vi "Phi Theta Scanning w Action Engine.vi"() -> ()   [LabVIEW 2022 SP3]
uses:
  C:/Users/mnopl/OneDrive/Documents/PhiThetaScanning/Thorlabs.MotionControl.Controls.dll
  Thorlabs.MotionControl.Controls.dll
  ActionEngineEnum.ctl
  <vilib>/DAQmx/read.llb/DAQmx Read (Analog 1D DBL 1Chan NSamp).vi
  <vilib>/Analysis/baseanly.llb/Mean (DBL).vi
  <vilib>/DAQmx/read.llb/DAQmx Read (Analog 2D DBL NChan NSamp).vi
  <vilib>/DAQmx/miscellaneous.llb/DAQmx Fill In Error Info.vi
  <vilib>/Analysis/NI_AALBase.lvlib
panel:
  out "Time Left":dbl
  out "X Origin":dbl
  out "Y Origin":dbl
  in  "Move to Origin":bool
  in  "Notes":string
  in  "X Center":dbl
  in  "Y Center":dbl
  in  "Tab Control 2":enum32{"Input 1", "Input 2"}(tab)
  out "Line Scan":dbl[](graph)
  in  "Save Line graph":bool
  out "Line Scan 2":dbl[](graph)
  in  "Save Line graph 2":bool
  in  "Duel Input":bool
  in  "Tab Control":enum32{"Input 1", "Input 2"}(tab)
  out "Graph":dbl[][](graph)
  in  "Save Image":bool
  in  "Save Data":bool
  in  "Name of File":string
  in  "Move to Cursor":bool
  in  "Save Image 2":bool
  out "Graph 2":dbl[][](graph)
  in  "Move to Cursor 2":bool
  in  "Estimate number\nof samples":bool
  in  "Connection":bool
  in  "Settings Y":T1={"Step Size (mm)"=10.0, "Initial Position"=0.0, "Move Absolute/Relative Position"=0.0, "Step Delay (ms)"=0, "Velocity (mm/s)"=0.0, "Acceleration (mm/s^2)"=0.0} {"Step Size (mm)" min=0.00046 format="%.8f"}
  in  "Settings X":T1={"Step Size (mm)"=10.0, "Initial Position"=0.0, "Move Absolute/Relative Position"=0.0, "Step Delay (ms)"=0, "Velocity (mm/s)"=0.0, "Acceleration (mm/s^2)"=0.0} {"Step Size (mm)" min=0.00046 format="%.8f"}
  in  "Estimate X Step Size":bool
  in  "2D Flyover":bool
  in  "Flyover Y Linescan":bool
  in  "Update Vel/Acc":bool
  in  "Grid points":dbl=3000.0
  in  "Save Phi/Theta":bool
  in  "Move to Saved Pos":bool
  in  "Save Position":bool
  out "Y Pos 1":dbl
  out "X Pos 1":dbl
  out "return value":dbl[][](array[numeric])
  in  "Acceleration":dbl=10.0
  in  "Measures/Pixel":dbl=7.0
  in  "Flyover X Linescan":bool
  in  "Move Y":bool
  in  "Move X":bool
  in  "Y Step Size":dbl=1.0
  in  "X Step Size":dbl=1.0
  in  "Move to Y":bool
  in  "Move to X":bool
  in  "Y Move":dbl=1.0
  in  "X Move":dbl=1.0
  out "Y Line Scan":dbl[](array[numeric])=[-inf, -inf, -inf, -inf, -inf, -inf]
  out "X Line Scan":dbl[](array[numeric])=[-inf, -inf, -inf, -inf, -inf, -inf]
  out "Scan Type":string="Scan"
  in  "Y Line Scan":bool
  in  "Abort":bool
  in  "X Line Scan":bool
  out "(X,Y)":cluster{dbl, dbl}[][](array[cluster])
  out "Phi Theta Data":dbl[][](graph)
  in  "Convert to phi/theta":bool
  in  "Y Pos":dbl=0.899996795693412
  in  "X Pos":dbl=1.0
  in  "Read Position":bool
  out "array of values":dbl[][](array[numeric])=[[-inf, -inf, -inf, -inf, -inf, -inf], [-inf, -inf, -inf, -inf, -inf, -inf], [-inf, -inf, -inf, -inf, -inf, -inf], [-inf, -inf, -inf, -inf, -inf, -inf], [-inf, -inf, -inf, -inf, -inf, -inf], [-inf, -inf, -inf, -inf, -inf, -inf]]
  out "task out":refnum<k21>
  in  "physical channels":tag="Dev1/ai0"
  in  "number of samples":i32=10000
  in  "rate":dbl=250000.0
  in  "maximum value":dbl=5.0 format="%0.2f"
  in  "minimum value":dbl=-5.0 format="%0.2f"
  in  "Take Single Measurement":bool
  out "Done Mov?":bool=TRUE
  in  "Y Length":dbl=5.0
  in  "X Length":dbl=5.0
  in  "2D Scan":bool
  in  "Velocity":dbl=2.0
  in  "Move Y (in)":bool
  in  "Move X (in)":bool
  in  "Time to wait":dbl=251.0
  out "Time":i32=77055304
  in  "Y Step Size (in)":dbl=1.0
  in  "X Step Size (in)":dbl=1.0
  in  "X=T,Y=F":bool
  in  "Moving?":bool
  in  "Stop":bool
  in  "KCubeStepperControl Y":refnum<k24>(container)
  in  "KCubeStepperControl X":refnum<k24>(container)
  in  "SerialNumber X":string="26005279"
  in  "SerialNumber Y":string="26005327"
  in  "Set Vel/Acc":bool
  out "array of values 2":dbl[][](array[numeric])
  # "Internal Variables"
  # "Only works with the first input"
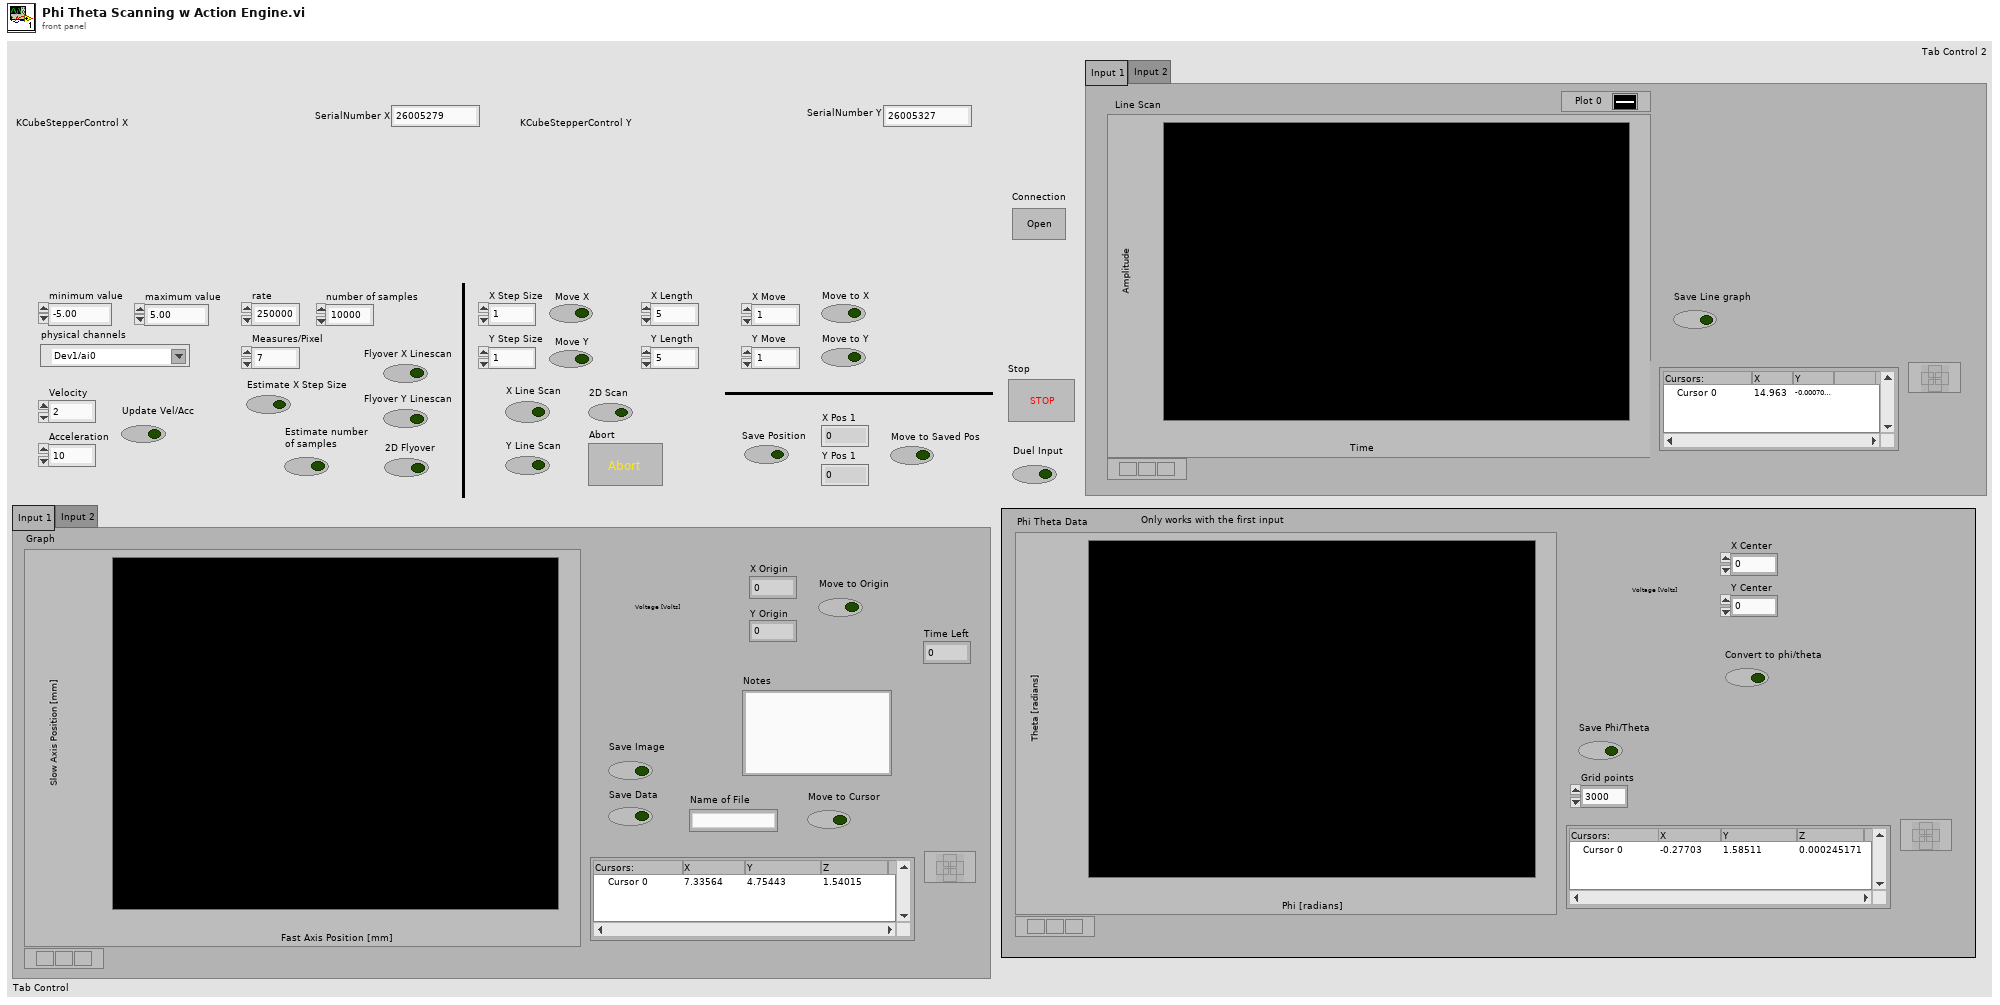
[diagram p1: front panel]
types:
  T1 = cluster{"Step Size (mm)":sgl, "Initial Position":dbl, "Move Absolute/Relative Position":dbl, "Step Delay (ms)":u32, "Velocity (mm/s)":dbl, "Acceleration (mm/s^2)":dbl}
  T2 = typedef "ActionEngineEnum.ctl" = enum16{"Open Connection", "Done", "Get Position", "Settings", "Home", "Move Absolute", "Move Relative", "Step", "Stop Action", "Close Connection"}
  T3 = typedef "LVPointDoubleTypeDef.ctl" = cluster{"Cursor X":dbl, "Cursor Y":dbl}
  T4 = typedef "imagedata.ctl" = cluster{"image type":i32, "image depth":i32, "image":u8[], "mask":u8[], "colors":u32[], "Rectangle":cluster{"left":i16, "top":i16, "right":i16, "bottom":i16}}
  T5 = cluster{"Y Step Size (in)":dbl, "Initial Position":dbl, "Move Absolute/Relative Position":dbl, "Step Delay (ms)":u32, "Velocity (mm/s)":dbl, "Acceleration (mm/s^2)":dbl}
  T6 = cluster{"X Step Size (in)":dbl, "Initial Position":dbl, "Move Absolute/Relative Position":dbl, "Step Delay (ms)":u32, "Velocity (mm/s)":dbl, "Acceleration (mm/s^2)":dbl}
  T7 = cluster{"Step Size (mm)":sgl, "Initial Position":dbl, "Move Absolute/Relative Position":dbl, "Step Delay (ms)":u32, "Velocity":dbl, "Acceleration":dbl}
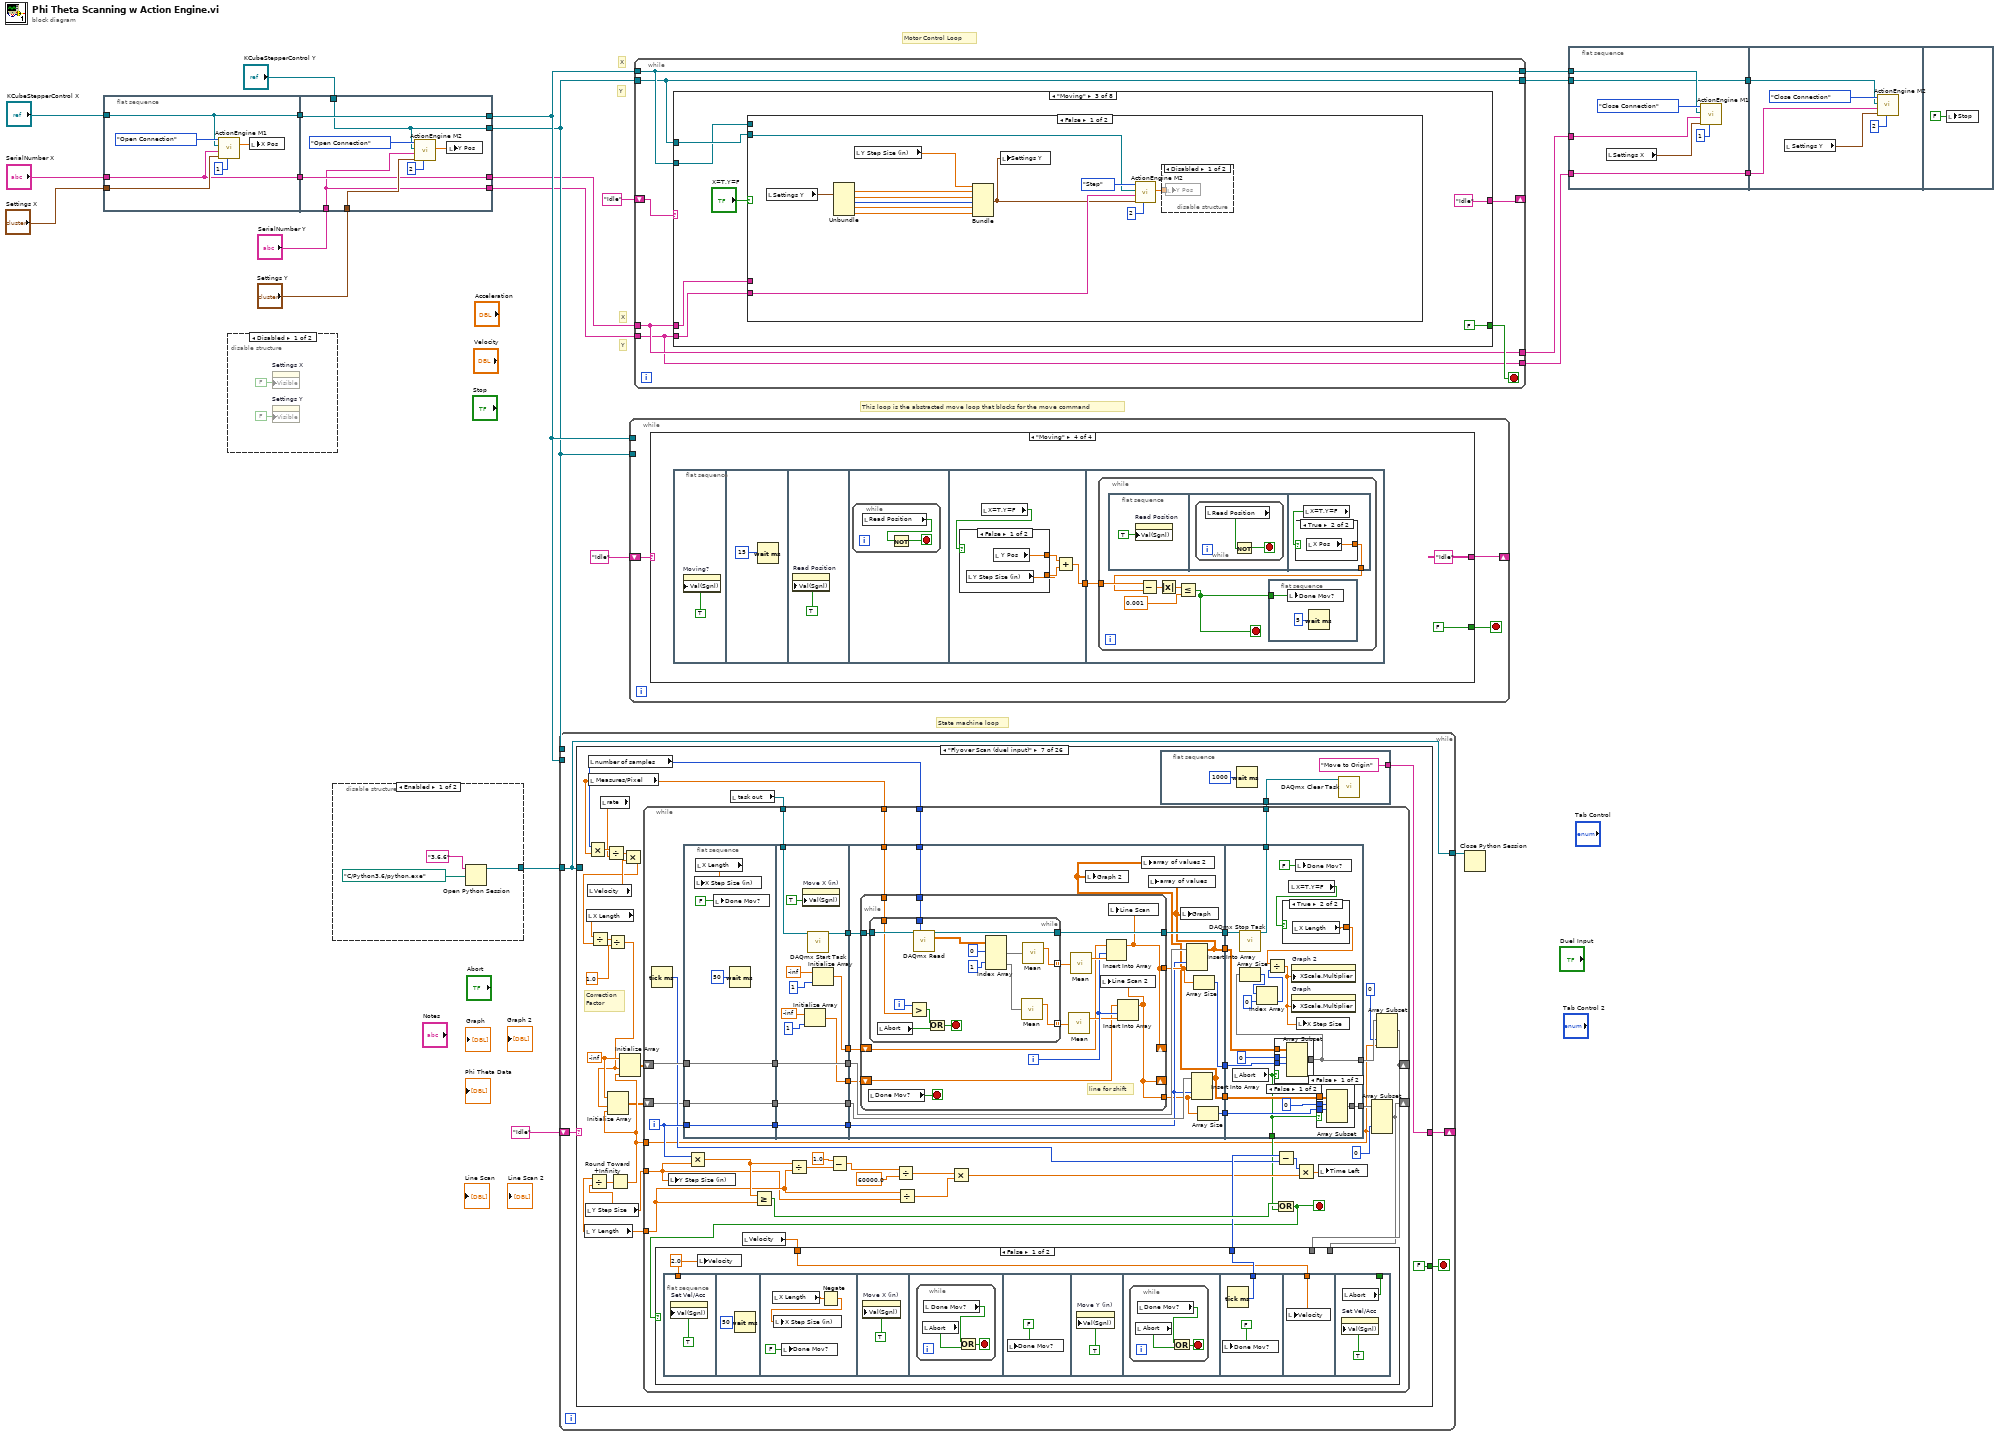
[diagram p0: block diagram]
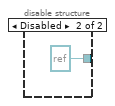
[diagram p3: hidden frame]
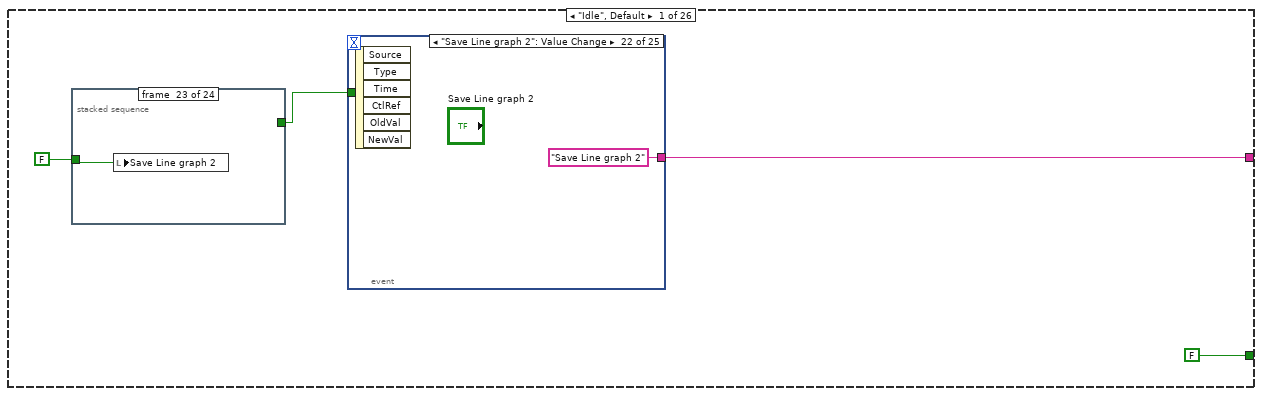
[diagram p4: hidden frame]
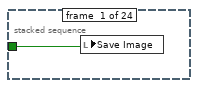
[diagram p5: hidden frame]
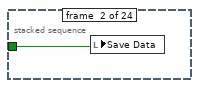
[diagram p6: hidden frame]
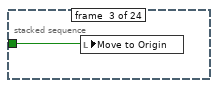
[diagram p7: hidden frame]
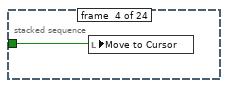
[diagram p8: hidden frame]
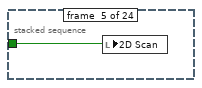
[diagram p9: hidden frame]
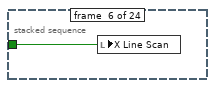
[diagram p10: hidden frame]
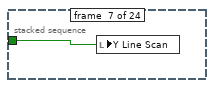
[diagram p11: hidden frame]
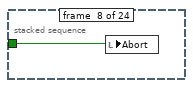
[diagram p12: hidden frame]
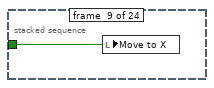
[diagram p13: hidden frame]
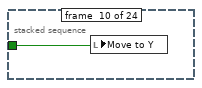
[diagram p14: hidden frame]
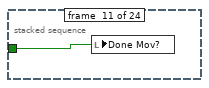
[diagram p15: hidden frame]
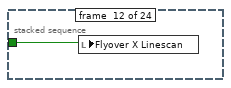
[diagram p16: hidden frame]
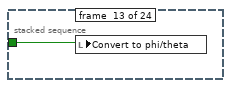
[diagram p17: hidden frame]
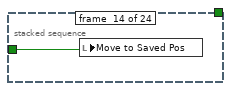
[diagram p18: hidden frame]
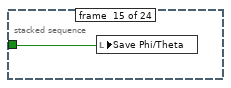
[diagram p19: hidden frame]
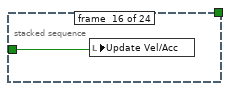
[diagram p20: hidden frame]
diagram:
  # "Y"
  # "X"
  # "State machine loop"
  # "Y"
  # "X"
  # "This loop is the abstracted move loop that blocks for the move command"
  # "Motor Control Loop"
  n1 = flat-sequence {
    tunnel: "SerialNumber X" -> [w24]
    tunnel: "Settings X" -> [w27]
    tunnel: "KCubeStepperControl X" -> [w25]
    tunnel: [w25] -> w10
    tunnel: [w24] -> w9
    tunnel: "SerialNumber Y" -> [w30]
    tunnel: "Settings Y" -> [w35]
    tunnel: "KCubeStepperControl Y" -> [w32]
    tunnel: w10 -> [w33]
    tunnel: w9 -> [w31]
    tunnel: [w33] -> w18
    tunnel: [w32] -> w17
    tunnel: [w31] -> w15
    tunnel: [w30] -> w16
    frame #0 {
      n2 = call "ActionEngine M1.vi"("ChannelNumber"=1, "Settings"=w27, "SerialNumber"=w24, "KCubeStepperControl"=w25, "Action"=ActionEngineEnum."Open Connection") -> ("Current Position"=w26:dbl)  [unwired: 4 in, 1 out]
      n3 = local write "X Pos"(w26) -> ()
    }
    frame #1 {
      n4 = call "ActionEngine M2.vi"("ChannelNumber"=2, "Settings"=w35, "SerialNumber"=w30, "KCubeStepperControl"=w32, "Action"=ActionEngineEnum."Open Connection") -> ("Current Position"=w34:dbl)  [unwired: 4 in, 1 out]
      n5 = local write "Y Pos"(w34) -> ()
    }
  }
  n6 = disable-structure shown="Disabled" {
    frame Disabled {
      n7 = property on="Settings X" class="Clust (strict)"("Visible"=FALSE) -> ()  [unwired: 2 in, 2 out]
      n8 = property on="Settings Y" class="Clust (strict)"("Visible"=FALSE) -> ()  [unwired: 2 in, 2 out]
    }
    frame Enabled {
    }
  }
  n9 = disable-structure shown="Enabled" {
    disable-tunnel: [w42 refnum<k35> refnum ("session out")] -> w20
    frame Enabled {
      n10 = Open Python Session(python version="3.6.6" ("Python version"), python path=path "C:/Python3.6/python.exe" ("Python path")) -> (session out=w42:refnum<k35>)  [unwired: 1 in, 1 out]
    }
    frame Disabled {
    }
  }
  n11 = while {
    shift-right: [w46] -> _
    shift-left: "Idle" -> [w47]
    tunnel: w20 -> [w44]
    tunnel: [w44] -> w19
    tunnel: w18 -> [_]
    tunnel: w17 -> [_]
    stop <- w45 stop-if-true
    n12 = case shown="\"Flyover Scan (duel input)\"" w47 {
      tunnel: [w51 "Init Graph" "Init Graph" ("Scan Type") w176 "Move to Origin" w543 w692 "Idle" ("Scan Type") "Idle" ("Scan Type") "Move to Origin" ("Scan Type") "Move to Origin" ("Scan Type") "Idle" ("Scan Type") "Idle" ("Scan Type") "Idle" "Idle" "Idle" ("Scan Type") "Idle" ("Scan Type") "Idle" "Idle" ("Scan Type") "Idle" "Idle" "Idle" ("Scan Type") "Idle" ("Scan Type") "Idle" ("Scan Type") "Idle" ("Scan Type") "Idle"] -> w46
      tunnel: [FALSE FALSE FALSE FALSE FALSE FALSE FALSE FALSE FALSE FALSE FALSE FALSE FALSE FALSE FALSE FALSE FALSE FALSE FALSE FALSE FALSE FALSE FALSE FALSE FALSE TRUE] -> w45
      tunnel: w44 -> [_ _ _ _ _ _ _ _ _ _ _ _ _ _ _ _ _ w1203 _ _ _ w1378 _ _ _ _]
      frame "Idle", Default {
        n13 = stacked-sequence {
          tunnel: FALSE -> [w52 w53 w54 w55 w56 w57 w58 w59 w60 w61 w62 w63 w64 w65 w66 w67 w68 w69 w70 w71 w72 w73 w74 w75]
          tunnel: [_ _ _ _ _ _ _ _ _ _ _ _ _ _ _ _ _ _ _ _ _ _ _ w75] -> w48
          frame #0 {
            n14 = local write "Save Image"(w52) -> ()
          }
          frame #1 {
            n15 = local write "Save Data"(w53) -> ()
          }
          frame #2 {
            n16 = local write "Move to Origin"(w54) -> ()
          }
          frame #3 {
            n17 = local write "Move to Cursor"(w55) -> ()
          }
          frame #4 {
            n18 = local write "2D Scan"(w56) -> ()
          }
          frame #5 {
            n19 = local write "X Line Scan"(w57) -> ()
          }
          frame #6 {
            n20 = local write "Y Line Scan"(w58) -> ()
          }
          frame #7 {
            n21 = local write "Abort"(w59) -> ()
          }
          frame #8 {
            n22 = local write "Move to X"(w60) -> ()
          }
          frame #9 {
            n23 = local write "Move to Y"(w61) -> ()
          }
          frame #10 {
            n24 = local write "Done Mov?"(w62) -> ()
          }
          frame #11 {
            n25 = local write "Flyover X Linescan"(w63) -> ()
          }
          frame #12 {
            n26 = local write "Convert to phi/theta"(w64) -> ()
          }
          frame #13 {
            n27 = local write "Move to Saved Pos"(w65) -> ()
          }
          frame #14 {
            n28 = local write "Save Phi/Theta"(w66) -> ()
          }
          frame #15 {
            n29 = local write "Update Vel/Acc"(w67) -> ()
          }
          frame #16 {
            n30 = local write "Flyover Y Linescan"(w68) -> ()
          }
          frame #17 {
            n31 = local write "2D Flyover"(w69) -> ()
          }
          frame #18 {
            n32 = local write "Estimate X Step Size"(w70) -> ()
          }
          frame #19 {
            n33 = local write "Estimate number\nof samples"(w71) -> ()
          }
          frame #20 {
            n34 = local write "Move to Cursor 2"(w72) -> ()
          }
          frame #21 {
            n35 = local write "Save Image 2"(w73) -> ()
          }
          frame #22 {
            n36 = local write "Save Line graph 2"(w74) -> ()
          }
          frame #23 {
            n37 = local write "Save Position"(w75) -> ()
          }
        }
        n38 = event shown="[21] \"Save Line graph 2\": Value Change" {
          selector: _ -> [_ _ _ _ _ _ _ _ _ _ _ _ _ _ _ _ _ _ _ _ _ _ _ _ _]
          dyn-events: _ -> [_ _ _ _ _ _ _ _ _ _ _ _ _ _ _ _ _ _ _ _ _ _ _ _ _]
          timeout: _ -> [_ _ _ _ _ _ _ _ _ _ _ _ _ _ _ _ _ _ _ _ _ _ _ _ _]
          tunnel: ["Idle" "Convert" "Move to Cursor" "Move to Cursor 2" "Stop" "Init Daq" "Init Daq (duel input)" "Move to Origin" "Move to Saved Position" "Init Daq" "Init Daq" "Init Daq" "Init Daq" "Move to" "Move to" "Update Vel/Acc" "Save Position" "Save Image" "Save Image 2" "Save Phi/Theta" "Save Line graph" "Save Line graph 2" "Save Data" "Estimate X Step Size" "Estimate number of samples"] -> w51
          tunnel: w48 -> [_ _ _ _ _ _ _ _ _ _ _ _ _ _ _ _ _ _ _ _ _ _ _ _ _]
          event Timeout {
            n39 = event-data() -> ()  [unwired: 1 in, 3 out]
          }
          event "Convert to phi/theta": Value Change {
            n40 = event-data() -> ()  [unwired: 1 in, 6 out]
          }
          event "Move to Cursor": Value Change {
            n41 = event-data() -> ()  [unwired: 1 in, 6 out]
          }
          event "Move to Cursor 2": Value Change {
            n42 = event-data() -> ()  [unwired: 1 in, 6 out]
          }
          event "Stop": Value Change {
            n43 = event-data() -> ()  [unwired: 1 in, 6 out]
          }
          event "2D Scan": Value Change {
            n44 = event-data() -> ()  [unwired: 1 in, 6 out]
            n45 = local read "X Step Size"() -> (w81:dbl)
            n46 = local read "Y Step Size"() -> (w82:dbl)
            n47 = local write "Scan Type"("Scan" ("Scan Type")) -> ()
            n48 = local write "Y Step Size (in)"(w82) -> ()
            n49 = local write "X Step Size (in)"(w81) -> ()
          }
          event "2D Flyover": Value Change {
            n50 = event-data() -> ()  [unwired: 1 in, 6 out]
            n51 = local read "Y Step Size"() -> (w87:dbl)
            n52 = local read "X Step Size"() -> (w88:dbl)
            n53 = local write "X Step Size (in)"(w88) -> ()
            n54 = local write "Y Step Size (in)"(w87) -> ()
            n55 = local write "Scan Type"("Flyover Scan (duel input)" ("Scan Type")) -> ()
          }
          event "Move to Origin": Value Change {
            n56 = event-data() -> ()  [unwired: 1 in, 6 out]
          }
          event "Move to Saved Pos": Value Change {
            n57 = event-data() -> ()  [unwired: 1 in, 6 out]
          }
          event "X Line Scan": Value Change {
            n58 = event-data() -> ()  [unwired: 1 in, 6 out]
            n59 = local read "X Step Size"() -> (w91:dbl)
            n60 = local write "X Step Size (in)"(w91) -> ()
            n61 = local write "Scan Type"("Line Scan" ("Scan Type")) -> ()
            n62 = local write "X=T,Y=F"(TRUE ("X=T,Y=F")) -> ()
          }
          event "Flyover X Linescan": Value Change {
            n63 = event-data() -> ()  [unwired: 1 in, 6 out]
            n64 = local read "X Step Size"() -> (w98:dbl)
            n65 = local write "X Step Size (in)"(w98) -> ()
            n66 = local write "Scan Type"("Flyover Linescan" ("Scan Type")) -> ()
            n67 = local write "X=T,Y=F"(TRUE ("X=T,Y=F")) -> ()
          }
          event "Flyover Y Linescan": Value Change {
            n68 = event-data() -> ()  [unwired: 1 in, 6 out]
            n69 = local read "Y Step Size"() -> (w100:dbl)
            n70 = local write "Y Step Size (in)"(w100) -> ()
            n71 = local write "Scan Type"("Flyover Linescan" ("Scan Type")) -> ()
            n72 = local write "X=T,Y=F"(FALSE ("X=T,Y=F")) -> ()
          }
          event "Y Line Scan": Value Change {
            n73 = event-data() -> ()  [unwired: 1 in, 6 out]
            n74 = local read "Y Step Size"() -> (w103:dbl)
            n75 = local write "Y Step Size (in)"(w103) -> ()
            n76 = local write "X=T,Y=F"(FALSE ("X=T,Y=F")) -> ()
            "Scan Type" <- "Line Scan" ("Scan Type")
          }
          event "Move to X": Value Change {
            n77 = event-data() -> ()  [unwired: 1 in, 6 out]
            n78 = local write "X=T,Y=F"(TRUE ("X=T,Y=F")) -> ()
          }
          event "Move to Y": Value Change {
            n79 = event-data() -> ()  [unwired: 1 in, 6 out]
            n80 = local write "X=T,Y=F"(FALSE ("X=T,Y=F")) -> ()
          }
          event "Update Vel/Acc": Value Change {
            n81 = event-data() -> ()  [unwired: 1 in, 6 out]
          }
          event "Save Position": Value Change {
            n82 = event-data() -> ()  [unwired: 1 in, 6 out]
          }
          event "Save Image": Value Change {
            n83 = event-data() -> ()  [unwired: 1 in, 6 out]
          }
          event "Save Image 2": Value Change {
            n84 = event-data() -> ()  [unwired: 1 in, 6 out]
          }
          event "Save Phi/Theta": Value Change {
            n85 = event-data() -> ()  [unwired: 1 in, 6 out]
          }
          event "Save Line graph": Value Change {
            n86 = event-data() -> ()  [unwired: 1 in, 6 out]
          }
          event "Save Line graph 2": Value Change {
            n87 = event-data() -> ()  [unwired: 1 in, 6 out]
          }
          event "Save Data": Value Change {
            n88 = event-data() -> ()  [unwired: 1 in, 6 out]
          }
          event "Estimate X Step Size": Value Change {
            n89 = event-data() -> ()  [unwired: 1 in, 6 out]
          }
          event "Estimate number\nof samples": Value Change {
            n90 = event-data() -> ()  [unwired: 1 in, 6 out]
          }
        }
      }
      frame "Init Daq" {
        w121 = -inf
        n91 = local read "Y Length"() -> (w134:dbl)
        n92 = local read "Y Step Size"() -> (w133:dbl)
        n93 = local read "X Length"() -> (w131:dbl)
        n94 = local read "X Step Size"() -> (w130:dbl)
        n95 = Divide(x=w134, y=w133) -> (x/y=w135:dbl)
        n96 = Divide(x=w131, y=w130) -> (x/y=w132:dbl)
        n97 = Round Toward +Infinity(x=w135) -> (ceil(x): smallest int >= x=w124:dbl)
        n98 = Round Toward +Infinity(x=w132) -> (ceil(x): smallest int >= x=w129:dbl)
        n99 = Increment(x=w124) -> (x+1=w122:dbl)
        n100 = Increment(x=w129) -> (x+1=w123:dbl)
        n101 = call "Initialize DAQ Assistant.vi"("minimum value"="minimum value", "maximum value"="maximum value", "rate"="rate", "number of samples"="number of samples", "physical channels"="physical channels") -> ("task out"=→"task out":refnum<k21>)  [unwired: 5 in, 1 out]
        n102 = Initialize Array(w121, w122) -> (→"Y Line Scan":dbl[])
        n103 = Initialize Array(w121, w123, w122) -> (→"array of values":dbl[][])
        n104 = Initialize Array(w121, w123) -> (→"X Line Scan":dbl[])
      }
      frame "Init Daq (duel input)" {
        w146 = -inf
        n105 = local read "Y Step Size"() -> (w158:dbl)
        n106 = local read "X Step Size"() -> (w161:dbl)
        n107 = local read "Y Length"() -> (w157:dbl)
        n108 = local read "X Length"() -> (w160:dbl)
        n109 = local read "number of samples"() -> (w149:i32)
        n110 = local read "physical channels"() -> (w150:tag)
        n111 = local read "maximum value"() -> (w151:dbl)
        n112 = local read "minimum value"() -> (w152:dbl)
        n113 = local read "rate"() -> (w148:dbl)
        n114 = Divide(x=w157, y=w158) -> (x/y=w156:dbl)
        n115 = Divide(x=w160, y=w161) -> (x/y=w159:dbl)
        n116 = Round Toward +Infinity(x=w156) -> (ceil(x): smallest int >= x=w163:dbl)
        n117 = Round Toward +Infinity(x=w159) -> (ceil(x): smallest int >= x=w162:dbl)
        n118 = Increment(x=w163) -> (x+1=w144:dbl)
        n119 = Increment(x=w162) -> (x+1=w145:dbl)
        n120 = call "Initialize DAQ Assistant (duel input).vi"("minimum value"=w152, "maximum value"=w151, "rate"=w148, "number of samples"=w149, "physical channels"=w150) -> ("task out"=w147:refnum<k21>)  [unwired: 5 in, 1 out]
        n121 = Initialize Array(w146, w145, w144) -> (→"array of values 2":dbl[][])
        n122 = Initialize Array(w146, w144) -> (w153:dbl[])
        n123 = Initialize Array(w146, w145, w144) -> (w154:dbl[][])
        n124 = Initialize Array(w146, w145) -> (w155:dbl[])
        n125 = local write "task out"(w147) -> ()
        n126 = local write "Y Line Scan"(w153) -> ()
        n127 = local write "array of values"(w154) -> ()
        n128 = local write "X Line Scan"(w155) -> ()
      }
      frame "Init Graph" {
        n129 = local read "Acceleration"() -> (w172:dbl)
        n130 = local read "Scan Type"() -> (w176:string)
        n131 = local read "Velocity"() -> (w173:dbl)
        n132 = flat-sequence {
          tunnel: [w261] -> w166
          tunnel: ["X Pos"] -> w178
          tunnel: ["Y Pos"] -> w177
          frame #0 {
            n133 = property on="Read Position" class="Bool (strict)"("Val(Sgnl)"=TRUE) -> ()  [unwired: 2 in, 2 out]
          }
          frame #1 {
            n134 = while {
              tunnel: [w262] -> w261
              stop <- w265 stop-if-true
              n135 = local read "Read Position"() -> (w264:bool)
              n136 = Not(x=w264) -> (.not. x?=w265:bool)
              n137 = Wait (ms)(milliseconds to wait=u32 10) -> (millisecond timer value=w262:u32)
            }
          }
          frame #2 {
            "X Origin" <- "X Pos"
            "Y Origin" <- "Y Pos"
          }
        }
        n138 = case shown="\"Flyover Scan\"" w176 {
          tunnel: [w194 w212 w228 w244] -> w170
          tunnel: w169 -> [w194 w212 w228 w244]
          frame "Line Scan", Default {
            n139 = local read "X=T,Y=F"() -> (w195:bool)
            n140 = case shown="False" w195 {
              frame False {
                n141 = flat-sequence {
                  frame #0 {
                    n142 = local read "Y Length"() -> (w197:dbl)
                    n143 = Divide(x=w197, y=2.0) -> (x/y=w198:dbl)
                    n144 = Negate(x=w198) -> (-x=w199:dbl)
                    n145 = local write "Y Step Size (in)"(w199) -> ()
                  }
                  frame #1 {
                    n146 = local write "Done Mov?"(FALSE ("Done Mov?")) -> ()
                    n147 = property on="Move Y (in)" class="Bool (strict)"("Val(Sgnl)"=TRUE ("Value (Signaling)")) -> ()  [unwired: 2 in, 2 out]
                  }
                  frame #2 {
                    n148 = while {
                      stop <- w202 stop-if-true
                      n149 = local read "Done Mov?"() -> (w202:bool)
                    }
                  }
                  frame #3 {
                    n150 = local write "Done Mov?"(FALSE ("Done Mov?")) -> ()
                  }
                }
              }
              frame True {
                n151 = flat-sequence {
                  frame #0 {
                    n152 = local read "X Length"() -> (w207:dbl)
                    n153 = Divide(x=w207, y=2.0) -> (x/y=w206:dbl)
                    n154 = Negate(x=w206) -> (-x=w205:dbl)
                    n155 = local write "X Step Size (in)"(w205) -> ()
                  }
                  frame #1 {
                    n156 = property on="Move X (in)" class="Bool (strict)"("Val(Sgnl)"=TRUE ("Value (Signaling)")) -> ()  [unwired: 2 in, 2 out]
                    n157 = local write "Done Mov?"(FALSE ("Done Mov?")) -> ()
                  }
                  frame #2 {
                    n158 = while {
                      stop <- w210 stop-if-true
                      n159 = local read "Done Mov?"() -> (w210:bool)
                    }
                  }
                  frame #3 {
                    n160 = local write "Done Mov?"(FALSE ("Done Mov?")) -> ()
                  }
                }
              }
            }
          }
          frame "Scan" {
            n161 = flat-sequence {
              frame #0 {
                n162 = local read "X Length"() -> (w220:dbl)
                n163 = local read "Y Length"() -> (w218:dbl)
                n164 = Divide(x=w220, y=2.0) -> (x/y=w216:dbl)
                n165 = Divide(x=w218, y=2.0) -> (x/y=w214:dbl)
                n166 = Negate(x=w216) -> (-x=w215:dbl)
                n167 = Negate(x=w214) -> (-x=w213:dbl)
                n168 = local write "X Step Size (in)"(w215) -> ()
                n169 = local write "Y Step Size (in)"(w213) -> ()
              }
              frame #1 {
                n170 = local write "Done Mov?"(FALSE ("Done Mov?")) -> ()
                n171 = property on="Move Y (in)" class="Bool (strict)"("Val(Sgnl)"=TRUE ("Value (Signaling)")) -> ()  [unwired: 2 in, 2 out]
              }
              frame #2 {
                n172 = while {
                  stop <- w223 stop-if-true
                  n173 = local read "Done Mov?"() -> (w223:bool)
                }
              }
              frame #3 {
                n174 = local write "Done Mov?"(FALSE ("Done Mov?")) -> ()
                n175 = property on="Move X (in)" class="Bool (strict)"("Val(Sgnl)"=TRUE ("Value (Signaling)")) -> ()  [unwired: 2 in, 2 out]
              }
              frame #4 {
                n176 = while {
                  stop <- w226 stop-if-true
                  n177 = local read "Done Mov?"() -> (w226:bool)
                }
              }
              frame #5 {
                n178 = local write "Done Mov?"(FALSE ("Done Mov?")) -> ()
              }
            }
          }
          frame "Flyover Scan" {
            n179 = flat-sequence {
              frame #0 {
                n180 = local read "X Length"() -> (w236:dbl)
                n181 = local read "Y Length"() -> (w234:dbl)
                n182 = Divide(x=w236, y=2.0) -> (x/y=w232:dbl)
                n183 = Divide(x=w234, y=2.0) -> (x/y=w230:dbl)
                n184 = Negate(x=w232) -> (-x=w231:dbl)
                n185 = Negate(x=w230) -> (-x=w229:dbl)
                n186 = local write "X Step Size (in)"(w231) -> ()
                n187 = local write "Y Step Size (in)"(w229) -> ()
              }
              frame #1 {
                n188 = local write "Done Mov?"(FALSE ("Done Mov?")) -> ()
                n189 = property on="Move Y (in)" class="Bool (strict)"("Val(Sgnl)"=TRUE ("Value (Signaling)")) -> ()  [unwired: 2 in, 2 out]
              }
              frame #2 {
                n190 = while {
                  stop <- w239 stop-if-true
                  n191 = local read "Done Mov?"() -> (w239:bool)
                }
              }
              frame #3 {
                n192 = local write "Done Mov?"(FALSE ("Done Mov?")) -> ()
                n193 = property on="Move X (in)" class="Bool (strict)"("Val(Sgnl)"=TRUE ("Value (Signaling)")) -> ()  [unwired: 2 in, 2 out]
              }
              frame #4 {
                n194 = while {
                  stop <- w242 stop-if-true
                  n195 = local read "Done Mov?"() -> (w242:bool)
                }
              }
              frame #5 {
                n196 = local write "Done Mov?"(FALSE ("Done Mov?")) -> ()
              }
            }
          }
          frame "Flyover Scan (duel input)" {
            n197 = flat-sequence {
              frame #0 {
                n198 = local read "X Length"() -> (w252:dbl)
                n199 = local read "Y Length"() -> (w250:dbl)
                n200 = Divide(x=w252, y=2.0) -> (x/y=w248:dbl)
                n201 = Divide(x=w250, y=2.0) -> (x/y=w246:dbl)
                n202 = Negate(x=w248) -> (-x=w247:dbl)
                n203 = Negate(x=w246) -> (-x=w245:dbl)
                n204 = local write "X Step Size (in)"(w247) -> ()
                n205 = local write "Y Step Size (in)"(w245) -> ()
              }
              frame #1 {
                n206 = local write "Done Mov?"(FALSE ("Done Mov?")) -> ()
                n207 = property on="Move Y (in)" class="Bool (strict)"("Val(Sgnl)"=TRUE ("Value (Signaling)")) -> ()  [unwired: 2 in, 2 out]
              }
              frame #2 {
                n208 = while {
                  stop <- w255 stop-if-true
                  n209 = local read "Done Mov?"() -> (w255:bool)
                }
              }
              frame #3 {
                n210 = local write "Done Mov?"(FALSE ("Done Mov?")) -> ()
                n211 = property on="Move X (in)" class="Bool (strict)"("Val(Sgnl)"=TRUE ("Value (Signaling)")) -> ()  [unwired: 2 in, 2 out]
              }
              frame #4 {
                n212 = while {
                  stop <- w258 stop-if-true
                  n213 = local read "Done Mov?"() -> (w258:bool)
                }
              }
              frame #5 {
                n214 = local write "Done Mov?"(FALSE ("Done Mov?")) -> ()
              }
            }
          }
        }
        n215 = flat-sequence {
          tunnel: w173 -> [w183]
          tunnel: [w183] -> w175
          tunnel: w172 -> [w180]
          tunnel: [w180] -> w174
          tunnel: w166 -> [_]
          tunnel: w175 -> [w186]
          tunnel: w174 -> [w185]
          tunnel: [w186] -> w168
          tunnel: [w185] -> w167
          tunnel: [w188] -> w169
          tunnel: [w189] -> w171
          tunnel: w168 -> [w189]
          tunnel: w167 -> [w188]
          frame #0 {
            n216 = local write "Acceleration"(10.0 ("Acceleration")) -> ()
            n217 = local write "Velocity"(2.0 ("Velocity")) -> ()
          }
          frame #1 {
            n218 = property on="Set Vel/Acc" class="Bool (strict)"("Val(Sgnl)"=TRUE ("Value (Signaling)")) -> ()  [unwired: 2 in, 2 out]
          }
          frame #2 {
            n219 = Wait (ms)(milliseconds to wait=u32 150) -> ()  [unwired: 1 out]
          }
        }
        n220 = case shown="\"Flyover Scan (duel input)\"" w176 {
          tunnel: w178 -> [w271 w290 w304 w316]
          tunnel: w177 -> [w270 w285 w300 w312]
          frame "Line Scan", Default {
            n221 = local read "X=T,Y=F"() -> (w269:bool)
            n222 = case shown="False" w269 {
              tunnel: w271 -> [_ w283]
              tunnel: w270 -> [w277 _]
              tunnel: [w272 w278] -> w268
              frame False {
                n223 = local read "Y Length"() -> (w275:dbl)
                n224 = local read "Y Step Size"() -> (w272:dbl)
                n225 = Divide(x=w275, y=2.0) -> (x/y=w273:dbl)
                n226 = Subtract(x=w277, y=w273) -> (x-y=w276:dbl)
                n227 = property on="Line Scan" class="WFGraph (strict)"("XScale.Offset"=w276) -> ()  [unwired: 2 in, 2 out]
              }
              frame True {
                n228 = local read "X Length"() -> (w281:dbl)
                n229 = Divide(x=w281, y=2.0) -> (x/y=w279:dbl)
                n230 = Subtract(x=w283, y=w279) -> (x-y=w282:dbl)
                n231 = local read "X Step Size"() -> (w278:dbl)
                n232 = property on="Line Scan" class="WFGraph (strict)"("XScale.Offset"=w282) -> ()  [unwired: 2 in, 2 out]
              }
            }
            n233 = property on="Line Scan" class="WFGraph (strict)"("XScale.Multiplier"=w268) -> ()  [unwired: 2 in, 2 out]
          }
          frame "Scan" {
            n234 = local read "X Length"() -> (w293:dbl)
            n235 = local read "Y Length"() -> (w288:dbl)
            n236 = Divide(x=w293, y=2.0) -> (x/y=w291:dbl)
            n237 = Divide(x=w288, y=2.0) -> (x/y=w286:dbl)
            n238 = local read "Y Step Size"() -> (w295:dbl)
            n239 = local read "X Step Size"() -> (w294:dbl)
            n240 = Subtract(x=w285, y=w286) -> (x-y=w284:dbl)
            n241 = Subtract(x=w290, y=w291) -> (x-y=w289:dbl)
            n242 = property on="Graph" class="IntGraph (strict)"("XScale.Offset"=w289) -> ()  [unwired: 2 in, 2 out]
            n243 = property on="Graph" class="IntGraph (strict)"("YScale.Offset"=w284) -> ()  [unwired: 2 in, 2 out]
            n244 = property on="Graph" class="IntGraph (strict)"("YScale.Multiplier"=w295) -> ()  [unwired: 2 in, 2 out]
            n245 = property on="Graph" class="IntGraph (strict)"("XScale.Multiplier"=w294) -> ()  [unwired: 2 in, 2 out]
          }
          frame "Flyover Scan" {
            n246 = local read "X Length"() -> (w307:dbl)
            n247 = local read "Y Length"() -> (w303:dbl)
            n248 = Divide(x=w307, y=2.0) -> (x/y=w305:dbl)
            n249 = Divide(x=w303, y=2.0) -> (x/y=w301:dbl)
            n250 = local read "X Step Size"() -> (w298:dbl)
            n251 = local read "Y Step Size"() -> (w296:dbl)
            n252 = Subtract(x=w300, y=w301) -> (x-y=w297:dbl)
            n253 = Subtract(x=w304, y=w305) -> (x-y=w299:dbl)
            n254 = property on="Graph" class="IntGraph (strict)"("YScale.Multiplier"=w296, "YScale.Offset"=w297) -> ()  [unwired: 2 in, 2 out]
            n255 = property on="Graph 2" class="IntGraph (strict)"("YScale.Multiplier"=w296, "YScale.Offset"=w297) -> ()  [unwired: 2 in, 2 out]
            n256 = property on="Graph" class="IntGraph (strict)"("XScale.Multiplier"=w298, "XScale.Offset"=w299) -> ()  [unwired: 2 in, 2 out]
            n257 = property on="Graph 2" class="IntGraph (strict)"("XScale.Multiplier"=w298, "XScale.Offset"=w299) -> ()  [unwired: 2 in, 2 out]
          }
          frame "Flyover Scan (duel input)" {
            n258 = local read "X Length"() -> (w319:dbl)
            n259 = local read "Y Length"() -> (w315:dbl)
            n260 = Divide(x=w319, y=2.0) -> (x/y=w317:dbl)
            n261 = Divide(x=w315, y=2.0) -> (x/y=w313:dbl)
            n262 = local read "X Step Size"() -> (w310:dbl)
            n263 = local read "Y Step Size"() -> (w308:dbl)
            n264 = Subtract(x=w312, y=w313) -> (x-y=w309:dbl)
            n265 = Subtract(x=w316, y=w317) -> (x-y=w311:dbl)
            n266 = property on="Graph" class="IntGraph (strict)"("YScale.Multiplier"=w308, "YScale.Offset"=w309) -> ()  [unwired: 2 in, 2 out]
            n267 = property on="Graph 2" class="IntGraph (strict)"("YScale.Multiplier"=w308, "YScale.Offset"=w309) -> ()  [unwired: 2 in, 2 out]
            n268 = property on="Graph" class="IntGraph (strict)"("XScale.Multiplier"=w310, "XScale.Offset"=w311) -> ()  [unwired: 2 in, 2 out]
            n269 = property on="Graph 2" class="IntGraph (strict)"("XScale.Multiplier"=w310, "XScale.Offset"=w311) -> ()  [unwired: 2 in, 2 out]
          }
        }
        n270 = flat-sequence {
          tunnel: w170 -> [w191]
          tunnel: w171 -> [w190]
          frame #0 {
            n271 = local write "Velocity"(w190) -> ()
            n272 = local write "Acceleration"(w191) -> ()
          }
          frame #1 {
            n273 = property on="Set Vel/Acc" class="Bool (strict)"("Val(Sgnl)"=TRUE ("Value (Signaling)")) -> ()  [unwired: 2 in, 2 out]
          }
          frame #2 {
            n274 = Wait (ms)(milliseconds to wait=u32 150) -> ()  [unwired: 1 out]
          }
        }
      }
      frame "Scan" {
        w327 = 0 ("Row")
        n275 = local read "number of samples"() -> (w323:i32)
        n276 = local read "Y Step Size"() -> (w321:dbl)
        n277 = local read "array of values"() -> (w325:dbl[][])
        n278 = local read "Y Origin"() -> (w332:dbl)
        n279 = local read "task out"() -> (w326:refnum<k21>)
        n280 = local read "X Origin"() -> (w334:dbl)
        n281 = local read "X Step Size"() -> (w338:dbl)
        n282 = Divide(x="Y Length", y=2.0) -> (x/y=w330:dbl)
        n283 = Divide(x="X Length", y=2.0) -> (x/y=w333:dbl)
        n284 = Divide(x="Y Length", y=w321) -> (x/y=w320:dbl)
        n285 = call "Measure and Update Array.vi"("Array In"=w325, "number of samples per channel"=w323, "task/channels in"=w326, "Row"=w327, "Column"=w327) -> ("Array Out"=w324:dbl[][])  [unwired: 7 in, 3 out]
        n286 = local write "Graph"(w324) -> ()
        n287 = Subtract(x=w332, y=w330) -> (x-y=w328:dbl)
        n288 = Subtract(x=w334, y=w333) -> (x-y=w329:dbl)
        n289 = while {
          shift-right: [w373] -> w340
          shift-left: w324 -> [w374]
          tunnel: [w369] -> w339 mode=indexing
          tunnel: "X Length" -> [w365]
          tunnel: w338 -> [w368]
          tunnel: w321 -> [w367]
          tunnel: "Y Length" -> [w366]
          tunnel: [w361] -> w337
          tunnel: "X Length" -> [w364]
          tunnel: w329 -> [w360]
          tunnel: w328 -> [w359]
          tunnel: w320 -> [w354]
          i -> [w371]
          stop <- w376 stop-if-true
          n290 = Multiply(x=w371, y=w367) -> (x*y=w370:dbl)
          n291 = while {
            tunnel: [w485] -> w363
            tunnel: w371 -> [w485]
            tunnel: [w484] -> w375
            shift-right: [w480] -> w347
            shift-left: w374 -> [w483]
            tunnel: [w482] -> w362
            tunnel: [w481] -> w372
            tunnel: w370 -> [w471]
            tunnel: [w479] -> w369 mode=indexing
            tunnel: w365 -> [w477]
            tunnel: w368 -> [w478]
            tunnel: w360 -> [w470]
            tunnel: w359 -> [w468]
            tunnel: [w466] -> w346
            i -> [w492]
            stop <- w489 stop-if-true
            n292 = flat-sequence {
              tunnel: w478 -> [w493]
              tunnel: w477 -> [w494]
              tunnel: w492 -> [w495]
              tunnel: [w495] -> w476
              tunnel: [w494] -> w475
              tunnel: [w493] -> w474
              tunnel: [w493] -> w467
              tunnel: [w505] -> w491
              tunnel: [w500] -> w486
              tunnel: [w496] -> w472
              tunnel: w476 -> [w498]
              tunnel: w475 -> [w502]
              tunnel: w474 -> [w501]
              tunnel: w467 -> [w497]
              tunnel: w491 -> [w508]
              tunnel: [w509] -> w490
              tunnel: [w511] -> w488
              tunnel: [w510] -> w487
              tunnel: w486 -> [w510]
              tunnel: [w506] -> w466
              tunnel: [w522] -> w489
              tunnel: w490 -> [w522]
              tunnel: w488 -> [_]
              tunnel: w487 -> [w515]
              tunnel: w485 -> [w520]
              tunnel: [w515] -> w484
              tunnel: [w519] -> w480
              tunnel: w483 -> [w518]
              tunnel: [w517] -> w482
              tunnel: [w516] -> w481
              frame #0 {
                n293 = local write "X Step Size (in)"(w493) -> ()
              }
              frame #1 {
                n294 = Increment(x=w498) -> (x+1=w500:i32)
                n295 = Multiply(x=w498, y=w497) -> (x*y=w496:dbl)
                n296 = local write "Done Mov?"(FALSE ("Done Moving?")) -> ()
                n297 = property on="Move X (in)" class="Bool (strict)"("Val(Sgnl)"=TRUE) -> ()  [unwired: 2 in, 2 out]
                n298 = Multiply(x=w501, y=w500) -> (x*y=w504:dbl)
                n299 = Less Or Equal?(x=w502, y=w504) -> (x <= y?=w505:bool)
              }
              frame #2 {
                n300 = while {
                  tunnel: [w513] -> w511
                  tunnel: [w512] -> w507
                  tunnel: [w512] -> w506
                  stop <- w514 stop-if-true
                  n301 = local read "Done Mov?"() -> (w513:bool)
                  n302 = local read "Abort"() -> (w512:bool)
                  n303 = Or(x=w513, y=w512) -> (x .or. y?=w514:bool)
                }
                n304 = Or(x=w508, y=w507) -> (x .or. y?=w509:bool)
              }
              frame #3 {
                n305 = local read "number of samples"() -> (w517:i32)
                n306 = local read "task out"() -> (w521:refnum<k21>)
                n307 = call "Measure and Update Array.vi"("Array In"=w518, "number of samples per channel"=w517, "task/channels in"=w521, "Row"=w515, "Column"=w520) -> ("Array Out"=w519:dbl[][], "task out"=w516:refnum<k21>)  [unwired: 7 in, 2 out]
              }
            }
            n308 = Add(x=w468, y=w471) -> (x+y=w469:dbl)
            n309 = Add(x=w472, y=w470) -> (x+y=w473:dbl)
            n310 = Bundle(w473, w469) -> (w479:cluster{dbl, dbl})  [unwired: 1 in]
            n311 = local write "Graph"(w480) -> ()
          }
          n312 = case shown="False" w346 {
            tunnel: [w390 TRUE] -> w376
            tunnel: w375 -> [w389 _]
            tunnel: [w388 w464] -> w373
            tunnel: w372 -> [w387 w463]
            tunnel: w367 -> [w386 _]
            tunnel: [w385 w463] -> w361
            tunnel: w366 -> [w384 _]
            tunnel: w364 -> [w383 _]
            tunnel: w363 -> [w382 _]
            tunnel: w347 -> [w381 w464]
            tunnel: w362 -> [w380 _]
            tunnel: [w378 w462] -> w357
            tunnel: [w377 1.0] -> w351
            frame False {
              n313 = flat-sequence {
                tunnel: w384 -> [w412]
                tunnel: w386 -> [w407]
                tunnel: w382 -> [w413]
                tunnel: [w413] -> w406
                tunnel: [w407] -> w405
                tunnel: [w412] -> w404
                tunnel: w383 -> [w411]
                tunnel: [TRUE ("Value (Signaling)")] -> w403
                tunnel: [w418] -> w402
                tunnel: [w417] -> w401
                tunnel: [w416] -> w400
                tunnel: w406 -> [w418]
                tunnel: w405 -> [w417]
                tunnel: w404 -> [w416]
                tunnel: w403 -> [w415]
                tunnel: [w414] -> w379
                tunnel: [w423] -> w399
                tunnel: [w421] -> w398
                tunnel: [w422] -> w397
                tunnel: w402 -> [w423]
                tunnel: w401 -> [w421]
                tunnel: w400 -> [w422]
                tunnel: [w420] -> w396
                tunnel: w379 -> [w419]
                tunnel: [w435] -> w395
                tunnel: [w430] -> w394
                tunnel: w399 -> [w431]
                tunnel: w398 -> [w433]
                tunnel: w397 -> [w428]
                tunnel: w396 -> [_]
                tunnel: [w427] -> w377
                tunnel: w395 -> [w438]
                tunnel: [w436] -> w393
                tunnel: [w440] -> w392
                tunnel: [w439] -> w391
                tunnel: w394 -> [w439]
                tunnel: [w445] -> w390
                tunnel: w393 -> [w445]
                tunnel: w392 -> [_]
                tunnel: w391 -> [w451]
                tunnel: w389 -> [_]
                tunnel: [w447] -> w388
                tunnel: w381 -> [w450]
                tunnel: w380 -> [w449]
                tunnel: w387 -> [w448]
                tunnel: [w446] -> w385
                tunnel: [w444] -> w378
                frame #0 {
                  n314 = Negate(x=w411) -> (-x=w409:dbl)
                  n315 = local write "X Step Size (in)"(w409) -> ()
                  n316 = local write "Y Step Size (in)"(w407) -> ()
                  n317 = local write "Done Mov?"(FALSE ("Done Moving?")) -> ()
                }
                frame #1 {
                  n318 = property on="Move X (in)" class="Bool (strict)"("Val(Sgnl)"=w415) -> (error out=w414:errorcluster)  [unwired: 2 in, 1 out]
                }
                frame #2 {
                  n319 = while {
                    tunnel: [w424] -> w420
                    tunnel: w419 -> [_]
                    stop <- w426 stop-if-true
                    n320 = local read "Done Mov?"() -> (w424:bool)
                    n321 = local read "Abort"() -> (w425:bool)
                    n322 = Or(x=w425, y=w424) -> (x .or. y?=w426:bool)
                  }
                }
                frame #3 {
                  n323 = local write "Done Mov?"(FALSE ("Done Mov?")) -> ()
                  n324 = property on="Move Y (in)" class="Bool (strict)"("Val(Sgnl)"=TRUE) -> ()  [unwired: 2 in, 2 out]
                  n325 = Multiply(x=w433, y=w431) -> (x*y=w429:dbl)
                  n326 = Increment(x=w431) -> (x+1=w430:i32)
                  n327 = Divide(x=w429, y=w428) -> (x/y=w427:dbl)
                  n328 = Less Or Equal?(x=w428, y=w429) -> (x <= y?=w435:bool)
                }
                frame #4 {
                  n329 = while {
                    tunnel: [w442] -> w440
                    tunnel: [w441] -> w437
                    stop <- w443 stop-if-true
                    n330 = local read "Done Mov?"() -> (w442:bool)
                    n331 = local read "Abort"() -> (w441:bool)
                    n332 = Or(x=w442, y=w441) -> (x .or. y?=w443:bool)
                  }
                  n333 = Or(x=w438, y=w437) -> (x .or. y?=w436:bool)
                }
                frame #5 {
                  n334 = case shown="False" w445 {
                    tunnel: w451 -> [w458 _]
                    tunnel: w450 -> [w457 w460]
                    tunnel: w449 -> [w456 _]
                    tunnel: w448 -> [w455 w459]
                    tunnel: [w454 w460] -> w447
                    tunnel: [w453 w459] -> w446
                    frame False {
                      n335 = call "Measure and Update Array.vi"("Array In"=w457, "number of samples per channel"=w456, "task/channels in"=w455, "Row"=0, "Column"=w458) -> ("Array Out"=w454:dbl[][], "task out"=w453:refnum<k21>)  [unwired: 7 in, 2 out]
                      n336 = local write "Graph"(w454) -> ()
                    }
                    frame True {
                    }
                  }
                  n337 = Tick Count (ms)() -> (millisecond timer value=w444:u32)
                }
              }
            }
            frame True {
              n338 = Tick Count (ms)() -> (millisecond timer value=w462:u32)
            }
          }
          n339 = Tick Count (ms)() -> (millisecond timer value=w358:u32)
          n340 = Subtract(x=1.0, y=w351) -> (x-y=w353:dbl)
          n341 = Subtract(x=w357, y=w358) -> (x-y=w356:u32)
          n342 = Multiply(x=w356, y=w353) -> (x*y=w355:dbl)
          n343 = Multiply(x=w355, y=w354) -> (x*y=w348:dbl)
          n344 = Divide(x=w348, y=60000.0) -> (x/y=→"Time Left":dbl)
        }
        n345 = local write "array of values"(w340) -> ()
        n346 = flat-sequence {
          tunnel: w339 -> [w345]
          frame #0 {
            n347 = local write "Done Mov?"(FALSE) -> ()
            n348 = Wait (ms)(milliseconds to wait=u32 2000) -> ()  [unwired: 1 out]
            "(X,Y)" <- w345
          }
        }
        n349 = call <vilib>:"DAQmx Clear Task.vi"("task in"=w337) -> ()  [unwired: 14 in, 1 out]
      }
      frame "Flyover Scan" {
        # "Correction\nFactor"
        n350 = local read "Y Length"() -> (w536:dbl)
        n351 = local read "Y Step Size"() -> (w537:dbl)
        n352 = local read "X Length"() -> (w527:dbl)
        n353 = local read "Velocity"() -> (w530:dbl)
        n354 = local read "number of samples"() -> (w535:i32)
        n355 = local read "Measures/Pixel"() -> (w534:dbl)
        n356 = Multiply(x=w535, y=w534) -> (x*y=w533:dbl)
        n357 = Divide(x=w536, y=w537) -> (x/y=w524:dbl)
        n358 = local read "rate"() -> (w532:dbl)
        n359 = Divide(x=w533, y=w532) -> (x/y=w531:dbl)
        n360 = Round Toward +Infinity(x=w524) -> (ceil(x): smallest int >= x=w523:dbl)
        n361 = Multiply(x=w531, y=w530) -> (x*y=w526:dbl)
        n362 = Divide(x=w527, y=w526) -> (x/y=w529:dbl)
        n363 = Divide(x=w529, y=1.0) -> (x/y=w528:dbl)
        n364 = Initialize Array(-inf, w528, w523) -> (w540:dbl[][])
        n365 = local read "task out"() -> (w539:refnum<k21>)
        n366 = while {
          shift-right: [w552] -> _
          shift-left: w540 -> [w579]
          tunnel: w537 -> [w554]
          tunnel: w536 -> [w555]
          tunnel: w539 -> [w572]
          tunnel: [w571] -> w538
          tunnel: w534 -> [w570]
          tunnel: w535 -> [w569]
          tunnel: w523 -> [w550]
          i -> [w575]
          stop <- w547 stop-if-true
          n367 = Tick Count (ms)() -> (millisecond timer value=w549:u32)
          n368 = local write "Y Step Size (in)"(w554) -> ()
          n369 = flat-sequence {
            tunnel: [w609] -> w580
            tunnel: w579 -> [w609]
            tunnel: [w608] -> w577
            tunnel: w575 -> [w608]
            tunnel: [w619] -> w581
            tunnel: w580 -> [w619]
            tunnel: [w617] -> w578
            tunnel: w577 -> [w617]
            tunnel: [w614] -> w576
            tunnel: [w613] -> w573
            tunnel: w572 -> [w612]
            tunnel: [w629] -> w583
            tunnel: [w623] -> w582
            tunnel: w581 -> [w626]
            tunnel: w578 -> [w620]
            tunnel: w576 -> [w628]
            tunnel: w573 -> [w627]
            tunnel: w570 -> [w625]
            tunnel: w569 -> [w624]
            tunnel: [w621] -> w561
            tunnel: w583 -> [w657]
            tunnel: w582 -> [w654]
            tunnel: [w651] -> w553
            tunnel: [w656] -> w571
            tunnel: w561 -> [w652]
            tunnel: [w650] -> w548
            frame #0 {
              n370 = local read "X Length"() -> (w610:dbl)
              n371 = local write "X Step Size (in)"(w610) -> ()
              n372 = local write "Done Mov?"(FALSE ("Done Moving?")) -> ()
              n373 = Wait (ms)(milliseconds to wait=u32 50) -> ()  [unwired: 1 out]
            }
            frame #1 {
              n374 = property on="Move X (in)" class="Bool (strict)"("Val(Sgnl)"=TRUE ("Value (Signaling)")) -> ()  [unwired: 2 in, 2 out]
              n375 = call <vilib>:"DAQmx Start Task.vi"("task/channels in"=w612) -> ("task out"=w613:refnum<k21>)  [unwired: 13 in, 1 out]
              n376 = Initialize Array(-inf, 1 ("dimension size")) -> (w614:dbl[])
            }
            frame #2 {
              n377 = while {
                tunnel: [w639] -> w629
                shift-right: [w633] -> _
                shift-left: w628 -> [w637]
                tunnel: w627 -> [w635]
                tunnel: [w633] -> w622
                tunnel: w625 -> [w632]
                tunnel: w624 -> [w631]
                i -> [w634]
                stop <- w630 stop-if-true
                n378 = while {
                  tunnel: w631 -> [w644]
                  tunnel: w635 -> [w647]
                  tunnel: [w646] -> w639
                  tunnel: w632 -> [w641]
                  tunnel: [w640] -> w638 mode=indexing
                  i -> [w643]
                  stop <- w649 stop-if-true
                  n379 = local read "Abort"() -> (w648:bool)
                  n380 = Greater?(x=w643, y=w641) -> (0:w642:bool)
                  n381 = Or(x=w642, y=w648) -> (x .or. y?=w649:bool)
                  n382 = call-poly <vilib>:"DAQmx Read.vi"("task/channels in"=w647, "number of samples per channel"=w644) -> ("task out"=w646:refnum<k21>, "data"=w645:dbl[])  [unwired: 11 in, 1 out]
                  n383 = call-poly <vilib>:"Mean.vi"("X"=w645) -> ("mean"=w640:dbl)  [unwired: 1 out]
                }
                n384 = local read "Done Mov?"() -> (w630:bool)
                n385 = call-poly <vilib>:"Mean.vi"("X"=w638) -> ("mean"=w636:dbl)  [unwired: 1 out]
                n386 = Insert Into Array(array=w637, index=w634, new element=w636) -> (w633:dbl[])
                n387 = local write "Line Scan"(w633) -> ()
              }
              n388 = Insert Into Array(array=w626, index (col)=w620, new element=w622) -> (w623:dbl[][])  [unwired: 1 in]
              n389 = local write "array of values"(w623) -> ()
              n390 = local write "Graph"(w623) -> ()
              n391 = Array Size(array=w622) -> (size(s)=w621:i32)
            }
            frame #3 {
              n392 = local read "Abort"() -> (w650:bool)
              n393 = call <vilib>:"DAQmx Stop Task.vi"("task/channels in"=w657) -> ("task out"=w656:refnum<k21>)  [unwired: 13 in, 1 out]
              n394 = case shown="False" w650 {
                tunnel: w654 -> [w667 w668]
                tunnel: 0 -> [w666 _]
                tunnel: w652 -> [w665 _]
                tunnel: [w664 w668] -> w651
                frame False {
                  n395 = Array Subset(array=w667, index (row)=w666, length (row)=w665) -> (w664:dbl[][])  [unwired: 2 in]
                }
                frame True {
                }
              }
              n396 = Array Size(array=w651) -> (size(s)=w660:i32[])
              n397 = Index Array(array=w660, index=0) -> (element=w658:i32)
              n398 = local read "X=T,Y=F"() -> (w662:bool)
              n399 = case shown="True" w662 {
                tunnel: [w669 w670] -> w661
                frame False {
                  n400 = local read "Y Length"() -> (w669:dbl)
                }
                frame True {
                  n401 = local read "X Length"() -> (w670:dbl)
                }
              }
              n402 = Divide(x=w661, y=w658) -> (x/y=w655:dbl)
              n403 = property on="Graph" class="IntGraph (strict)"("XScale.Multiplier"=w655) -> ()  [unwired: 2 in, 2 out]
              n404 = local write "Done Mov?"(FALSE ("Done Mov?")) -> ()
              n405 = local write "X Step Size"(w655) -> ()
            }
          }
          n406 = Multiply(x=w575, y=w554) -> (x*y=w560:dbl)
          n407 = local read "Velocity"() -> (w559:dbl)
          n408 = Greater Or Equal?(x=w560, y=w555) -> (x >= y?=w574:bool)
          n409 = Divide(x=w560, y=w555) -> (x/y=w568:dbl)
          n410 = Subtract(x=1.0, y=w568) -> (x-y=w563:dbl)
          n411 = Divide(x=w563, y=60000.0) -> (x/y=w558:dbl)
          n412 = Divide(x=w555, y=w554) -> (x/y=w556:dbl)
          n413 = Multiply(x=w558, y=w556) -> (x*y=w557:dbl)
          n414 = Or(x=w574, y=w548) -> (x .or. y?=w547:bool)
          n415 = Array Subset(array=w553, index (col)=0, length (col)=w550) -> (w552:dbl[][])  [unwired: 2 in]
          n416 = case shown="False" w547 {
            tunnel: w552 -> [_ _]
            tunnel: [w586 u32 0 ("millisecond timer value")] -> w566
            tunnel: w559 -> [w584 _]
            frame False {
              w585 = 2.0 ("Velocity")
              n417 = flat-sequence {
                tunnel: w585 -> [_]
                tunnel: [w601] -> w586
                tunnel: w584 -> [w603]
                tunnel: [w604] -> _
                frame #0 {
                  n418 = property on="Set Vel/Acc" class="Bool (strict)"("Val(Sgnl)"=TRUE ("Value (Signaling)")) -> ()  [unwired: 2 in, 2 out]
                }
                frame #1 {
                  n419 = Wait (ms)(milliseconds to wait=u32 50) -> ()  [unwired: 1 out]
                }
                frame #2 {
                  n420 = local read "X Length"() -> (w591:dbl)
                  n421 = local write "Done Mov?"(FALSE ("Done Mov?")) -> ()
                  n422 = Negate(x=w591) -> (-x=w590:dbl)
                  n423 = local write "X Step Size (in)"(w590) -> ()
                }
                frame #3 {
                  n424 = property on="Move X (in)" class="Bool (strict)"("Val(Sgnl)"=TRUE ("Value (Signaling)")) -> ()  [unwired: 2 in, 2 out]
                }
                frame #4 {
                  n425 = while {
                    stop <- w595 stop-if-true
                    n426 = local read "Abort"() -> (w593:bool)
                    n427 = local read "Done Mov?"() -> (w594:bool)
                    n428 = Or(x=w594, y=w593) -> (x .or. y?=w595:bool)
                  }
                }
                frame #5 {
                  n429 = local write "Done Mov?"(FALSE ("Done Mov?")) -> ()
                }
                frame #6 {
                  n430 = property on="Move Y (in)" class="Bool (strict)"("Val(Sgnl)"=TRUE ("Value (Signaling)")) -> ()  [unwired: 2 in, 2 out]
                }
                frame #7 {
                  n431 = while {
                    stop <- w600 stop-if-true
                    n432 = local read "Abort"() -> (w598:bool)
                    n433 = local read "Done Mov?"() -> (w599:bool)
                    n434 = Or(x=w599, y=w598) -> (x .or. y?=w600:bool)
                  }
                }
                frame #8 {
                  n435 = local write "Done Mov?"(FALSE ("Done Mov?")) -> ()
                  n436 = Tick Count (ms)() -> (millisecond timer value=w601:u32)
                }
                frame #9 {
                  n437 = local write "Velocity"(w603) -> ()
                }
                frame #10 {
                  n438 = property on="Set Vel/Acc" class="Bool (strict)"("Val(Sgnl)"=TRUE) -> ()  [unwired: 2 in, 2 out]
                  n439 = local read "Abort"() -> (w604:bool)
                }
              }
              n440 = local write "Velocity"(w585) -> ()
            }
            frame True {
            }
          }
          n441 = Subtract(x=w566, y=w549) -> (x-y=w565:u32)
          n442 = Multiply(x=w565, y=w557) -> (x*y=w564:dbl)
          n443 = local write "Time Left"(w564) -> ()
        }
        n444 = flat-sequence {
          tunnel: ["Move to Origin" ("Scan Type")] -> w543
          tunnel: w538 -> [w545]
          frame #0 {
            n445 = Wait (ms)(milliseconds to wait=u32 1000) -> ()  [unwired: 1 out]
            n446 = call <vilib>:"DAQmx Clear Task.vi"("task in"=w545) -> ()  [unwired: 14 in, 1 out]
          }
        }
      }
      frame "Flyover Scan (duel input)" {
        w674 = -inf
        # "Correction\nFactor"
        n447 = local read "Y Length"() -> (w687:dbl)
        n448 = local read "Y Step Size"() -> (w675:dbl)
        n449 = local read "X Length"() -> (w679:dbl)
        n450 = local read "Velocity"() -> (w681:dbl)
        n451 = local read "number of samples"() -> (w686:i32)
        n452 = local read "Measures/Pixel"() -> (w685:dbl)
        n453 = Multiply(x=w686, y=w685) -> (x*y=w684:dbl)
        n454 = Divide(x=w687, y=w675) -> (x/y=w676:dbl)
        n455 = local read "rate"() -> (w683:dbl)
        n456 = Divide(x=w684, y=w683) -> (x/y=w682:dbl)
        n457 = Round Toward +Infinity(x=w676) -> (ceil(x): smallest int >= x=w672:dbl)
        n458 = Multiply(x=w682, y=w681) -> (x*y=w678:dbl)
        n459 = Divide(x=w679, y=w678) -> (x/y=w680:dbl)
        n460 = Divide(x=w680, y=1.0) -> (x/y=w673:dbl)
        n461 = Initialize Array(w674, w673, w672) -> (w671:dbl[][])
        n462 = Initialize Array(w674, w673, w672) -> (w690:dbl[][])
        n463 = local read "task out"() -> (w689:refnum<k21>)
        n464 = while {
          shift-right: [w710] -> _
          shift-left: w690 -> [w737]
          tunnel: w675 -> [w712]
          tunnel: w687 -> [w713]
          tunnel: w689 -> [w730]
          tunnel: [w729] -> w688
          tunnel: w685 -> [w728]
          tunnel: w686 -> [w727]
          tunnel: w672 -> [w697]
          shift-right: [w696] -> _
          shift-left: w671 -> [w702]
          i -> [w733]
          stop <- w706 stop-if-true
          n465 = Tick Count (ms)() -> (millisecond timer value=w708:u32)
          n466 = local write "Y Step Size (in)"(w712) -> ()
          n467 = flat-sequence {
            tunnel: [w768] -> w738
            tunnel: w737 -> [w768]
            tunnel: [w767] -> w735
            tunnel: w733 -> [w767]
            tunnel: [w765] -> w703
            tunnel: w702 -> [w765]
            tunnel: [w782] -> w739
            tunnel: w738 -> [w782]
            tunnel: [w780] -> w736
            tunnel: w735 -> [w780]
            tunnel: [w777] -> w734
            tunnel: [w776] -> w731
            tunnel: w730 -> [w775]
            tunnel: [w772] -> w705
            tunnel: [w771] -> w704
            tunnel: w703 -> [w771]
            tunnel: [w797] -> w741
            tunnel: [w791] -> w740
            tunnel: w739 -> [w794]
            tunnel: w736 -> [w786]
            tunnel: w734 -> [w796]
            tunnel: w731 -> [w795]
            tunnel: w728 -> [w793]
            tunnel: w727 -> [w792]
            tunnel: [w789] -> w719
            tunnel: w705 -> [w788]
            tunnel: w704 -> [w787]
            tunnel: [w783] -> w701
            tunnel: [w784] -> w700
            tunnel: w741 -> [w838]
            tunnel: w740 -> [w836]
            tunnel: [w833] -> w711
            tunnel: [w837] -> w729
            tunnel: w719 -> [w834]
            tunnel: [w828] -> w707
            tunnel: w701 -> [w831]
            tunnel: w700 -> [w829]
            tunnel: [w827] -> w699
            frame #0 {
              n468 = local read "X Length"() -> (w769:dbl)
              n469 = local write "X Step Size (in)"(w769) -> ()
              n470 = local write "Done Mov?"(FALSE ("Done Moving?")) -> ()
              n471 = Wait (ms)(milliseconds to wait=u32 50) -> ()  [unwired: 1 out]
            }
            frame #1 {
              n472 = property on="Move X (in)" class="Bool (strict)"("Val(Sgnl)"=TRUE ("Value (Signaling)")) -> ()  [unwired: 2 in, 2 out]
              n473 = Initialize Array(-inf, 1 ("dimension size")) -> (w772:dbl[])
              n474 = call <vilib>:"DAQmx Start Task.vi"("task/channels in"=w775) -> ("task out"=w776:refnum<k21>)  [unwired: 13 in, 1 out]
              n475 = Initialize Array(-inf, 1 ("dimension size")) -> (w777:dbl[])
            }
            frame #2 {
              n476 = while {
                tunnel: [w811] -> w797
                shift-right: [w807] -> _
                shift-left: w796 -> [w800]
                tunnel: w795 -> [w808]
                tunnel: [w807] -> w790
                tunnel: w793 -> [w806]
                tunnel: w792 -> [w805]
                shift-right: [w798] -> _
                shift-left: w788 -> [w799]
                tunnel: [w798] -> w785
                i -> [w802]
                stop <- w804 stop-if-true
                # "line for shift"
                n477 = local read "Done Mov?"() -> (w804:bool)
                n478 = while {
                  tunnel: w805 -> [w822]
                  tunnel: w808 -> [w824]
                  tunnel: [w823] -> w811
                  tunnel: w806 -> [w819]
                  tunnel: [w818] -> w810 mode=indexing
                  tunnel: [w812] -> w803 mode=indexing
                  i -> [w821]
                  stop <- w826 stop-if-true
                  n479 = local read "Abort"() -> (w825:bool)
                  n480 = Greater?(x=w821, y=w819) -> (0:w820:bool)
                  n481 = call-poly <vilib>:"DAQmx Read.vi"("task/channels in"=w824, "number of samples per channel"=w822) -> ("task out"=w823:refnum<k21>, "data"=w817:dbl[][])  [unwired: 11 in, 1 out]
                  n482 = Or(x=w820, y=w825) -> (x .or. y?=w826:bool)
                  n483 = Index Array(array=w817, index (row) #1=0 ("index (row)"), index (row) #2=1 ("index (row)")) -> (element #1=w816:dbl[], element #2=w815:dbl[])  [unwired: 2 in]
                  n484 = call-poly <vilib>:"Mean.vi"("X"=w815) -> ("mean"=w812:dbl)  [unwired: 1 out]
                  n485 = call-poly <vilib>:"Mean.vi"("X"=w816) -> ("mean"=w818:dbl)  [unwired: 1 out]
                }
                n486 = call-poly <vilib>:"Mean.vi"("X"=w803) -> ("mean"=w801:dbl)  [unwired: 1 out]
                n487 = call-poly <vilib>:"Mean.vi"("X"=w810) -> ("mean"=w809:dbl)  [unwired: 1 out]
                n488 = Insert Into Array(array=w800, index=w802, new element=w809) -> (w807:dbl[])
                n489 = local write "Line Scan"(w807) -> ()
                n490 = Insert Into Array(array=w799, index=w802, new element=w801) -> (w798:dbl[])
                n491 = local write "Line Scan 2"(w798) -> ()
              }
              n492 = Insert Into Array(array=w794, index (col)=w786, new element=w790) -> (w791:dbl[][])  [unwired: 1 in]
              n493 = local write "array of values"(w791) -> ()
              n494 = local write "Graph"(w791) -> ()
              n495 = Insert Into Array(array=w787, index (col)=w786, new element=w785) -> (w783:dbl[][])  [unwired: 1 in]
              n496 = local write "Graph 2"(w783) -> ()
              n497 = local write "array of values 2"(w783) -> ()
              n498 = Array Size(array=w790) -> (size(s)=w789:i32)
              n499 = Array Size(array=w785) -> (size(s)=w784:i32)
            }
            frame #3 {
              n500 = local read "Abort"() -> (w828:bool)
              n501 = call <vilib>:"DAQmx Stop Task.vi"("task/channels in"=w838) -> ("task out"=w837:refnum<k21>)  [unwired: 13 in, 1 out]
              n502 = case shown="False" w828 {
                tunnel: w836 -> [w853 w854]
                tunnel: 0 -> [w852 _]
                tunnel: w834 -> [w851 _]
                tunnel: [w850 w854] -> w833
                frame False {
                  n503 = Array Subset(array=w853, index (row)=w852, length (row)=w851) -> (w850:dbl[][])  [unwired: 2 in]
                }
                frame True {
                }
              }
              n504 = Array Size(array=w833) -> (size(s)=w841:i32[])
              n505 = Index Array(array=w841, index=0) -> (element=w839:i32)
              n506 = local read "X=T,Y=F"() -> (w843:bool)
              n507 = case shown="True" w843 {
                tunnel: [w855 w856] -> w842
                frame False {
                  n508 = local read "Y Length"() -> (w855:dbl)
                }
                frame True {
                  n509 = local read "X Length"() -> (w856:dbl)
                }
              }
              n510 = Divide(x=w842, y=w839) -> (x/y=w832:dbl)
              n511 = property on="Graph 2" class="IntGraph (strict)"("XScale.Multiplier"=w832) -> ()  [unwired: 2 in, 2 out]
              n512 = property on="Graph" class="IntGraph (strict)"("XScale.Multiplier"=w832) -> ()  [unwired: 2 in, 2 out]
              n513 = local write "Done Mov?"(FALSE ("Done Mov?")) -> ()
              n514 = local write "X Step Size"(w832) -> ()
              n515 = case shown="False" w828 {
                tunnel: w831 -> [w848 w849]
                tunnel: 0 -> [w847 _]
                tunnel: w829 -> [w846 _]
                tunnel: [w845 w849] -> w827
                frame False {
                  n516 = Array Subset(array=w848, index (row)=w847, length (row)=w846) -> (w845:dbl[][])  [unwired: 2 in]
                }
                frame True {
                }
              }
            }
          }
          n517 = Multiply(x=w733, y=w712) -> (x*y=w718:dbl)
          n518 = local read "Velocity"() -> (w717:dbl)
          n519 = Greater Or Equal?(x=w718, y=w713) -> (x >= y?=w732:bool)
          n520 = Divide(x=w718, y=w713) -> (x/y=w726:dbl)
          n521 = Subtract(x=1.0, y=w726) -> (x-y=w721:dbl)
          n522 = Divide(x=w721, y=60000.0) -> (x/y=w716:dbl)
          n523 = Divide(x=w713, y=w712) -> (x/y=w714:dbl)
          n524 = Multiply(x=w716, y=w714) -> (x*y=w715:dbl)
          n525 = Or(x=w732, y=w707) -> (x .or. y?=w706:bool)
          n526 = Array Subset(array=w699, index (col)=0, length (col)=w697) -> (w696:dbl[][])  [unwired: 2 in]
          n527 = Array Subset(array=w711, index (col)=0, length (col)=w697) -> (w710:dbl[][])  [unwired: 2 in]
          n528 = case shown="False" w706 {
            tunnel: w710 -> [_ _]
            tunnel: [w744 u32 0 ("millisecond timer value")] -> w724
            tunnel: w717 -> [w742 _]
            tunnel: w696 -> [_ _]
            frame False {
              w743 = 2.0 ("Velocity")
              n529 = flat-sequence {
                tunnel: w743 -> [_]
                tunnel: [w759] -> w744
                tunnel: w742 -> [w761]
                tunnel: [w762] -> _
                frame #0 {
                  n530 = property on="Set Vel/Acc" class="Bool (strict)"("Val(Sgnl)"=TRUE ("Value (Signaling)")) -> ()  [unwired: 2 in, 2 out]
                }
                frame #1 {
                  n531 = Wait (ms)(milliseconds to wait=u32 50) -> ()  [unwired: 1 out]
                }
                frame #2 {
                  n532 = local read "X Length"() -> (w749:dbl)
                  n533 = local write "Done Mov?"(FALSE ("Done Mov?")) -> ()
                  n534 = Negate(x=w749) -> (-x=w748:dbl)
                  n535 = local write "X Step Size (in)"(w748) -> ()
                }
                frame #3 {
                  n536 = property on="Move X (in)" class="Bool (strict)"("Val(Sgnl)"=TRUE ("Value (Signaling)")) -> ()  [unwired: 2 in, 2 out]
                }
                frame #4 {
                  n537 = while {
                    stop <- w753 stop-if-true
                    n538 = local read "Abort"() -> (w751:bool)
                    n539 = local read "Done Mov?"() -> (w752:bool)
                    n540 = Or(x=w752, y=w751) -> (x .or. y?=w753:bool)
                  }
                }
                frame #5 {
                  n541 = local write "Done Mov?"(FALSE ("Done Mov?")) -> ()
                }
                frame #6 {
                  n542 = property on="Move Y (in)" class="Bool (strict)"("Val(Sgnl)"=TRUE ("Value (Signaling)")) -> ()  [unwired: 2 in, 2 out]
                }
                frame #7 {
                  n543 = while {
                    stop <- w758 stop-if-true
                    n544 = local read "Abort"() -> (w756:bool)
                    n545 = local read "Done Mov?"() -> (w757:bool)
                    n546 = Or(x=w757, y=w756) -> (x .or. y?=w758:bool)
                  }
                }
                frame #8 {
                  n547 = local write "Done Mov?"(FALSE ("Done Mov?")) -> ()
                  n548 = Tick Count (ms)() -> (millisecond timer value=w759:u32)
                }
                frame #9 {
                  n549 = local write "Velocity"(w761) -> ()
                }
                frame #10 {
                  n550 = property on="Set Vel/Acc" class="Bool (strict)"("Val(Sgnl)"=TRUE) -> ()  [unwired: 2 in, 2 out]
                  n551 = local read "Abort"() -> (w762:bool)
                }
              }
              n552 = local write "Velocity"(w743) -> ()
            }
            frame True {
            }
          }
          n553 = Subtract(x=w724, y=w708) -> (x-y=w723:u32)
          n554 = Multiply(x=w723, y=w715) -> (x*y=w722:dbl)
          n555 = local write "Time Left"(w722) -> ()
        }
        n556 = flat-sequence {
          tunnel: ["Move to Origin" ("Scan Type")] -> w692
          tunnel: w688 -> [w694]
          frame #0 {
            n557 = Wait (ms)(milliseconds to wait=u32 1000) -> ()  [unwired: 1 out]
            n558 = call <vilib>:"DAQmx Clear Task.vi"("task in"=w694) -> ()  [unwired: 14 in, 1 out]
          }
        }
      }
      frame "Estimate X Step Size" {
        # "Was initially 1"
        # "Correction Factor"
        n559 = local read "number of samples"() -> (w867:i32)
        n560 = local read "Measures/Pixel"() -> (w866:dbl)
        n561 = Multiply(x=w867, y=w866) -> (x*y=w864:dbl)
        n562 = local read "rate"() -> (w865:dbl)
        n563 = local read "Velocity"() -> (w863:dbl)
        n564 = Divide(x=w864, y=w865) -> (x/y=w862:dbl)
        n565 = Multiply(x=w863, y=w862) -> (x*y=w861:dbl)
        n566 = Multiply(x=w861, y=1.0 ("x*y")) -> (x*y=w860:dbl)
        n567 = local write "X Step Size"(w860) -> ()
      }
      frame "Estimate number of samples" {
        n568 = flat-sequence {
          tunnel: [w889] -> w868
          frame #0 {
            n569 = local write "Measures/Pixel"(7.0 ("Measures/Pixel")) -> ()
          }
          frame #1 {
            n570 = while {
              tunnel: [w890] -> w889
              stop <- w890 stop-if-true
              n571 = flat-sequence {
                tunnel: [w900] -> w892
                frame #0 {
                  n572 = local read "Measures/Pixel"() -> (w895:dbl)
                  n573 = local read "X Step Size"() -> (w894:dbl)
                  n574 = local read "Velocity"() -> (w896:dbl)
                  n575 = local read "rate"() -> (w893:dbl)
                  n576 = Multiply(x=w893, y=w894) -> (x*y=w897:dbl)
                  n577 = Multiply(x=w895, y=w896) -> (x*y=w898:dbl)
                  n578 = Divide(x=w897, y=w898) -> (x/y=w899:dbl)
                  n579 = local write "number of samples"(w899) -> ()
                }
                frame #1 {
                  n580 = local read "number of samples"() -> (w903:i32)
                  n581 = Greater?(x=w903, y=10000) -> (0:w902:bool)
                  n582 = case shown="True" w902 {
                    selector: w902 -> [w904 w908]
                    tunnel: [w904 w908] -> w900
                    frame False {
                    }
                    frame True {
                      n583 = local read "Measures/Pixel"() -> (w907:dbl)
                      n584 = Add(x=w907, y=4.0) -> (x+y=w905:dbl)
                      n585 = local write "Measures/Pixel"(w905) -> ()
                    }
                  }
                }
              }
              n586 = Wait (ms)(milliseconds to wait=u32 10) -> ()  [unwired: 1 out]
              n587 = Not(x=w892) -> (.not. x?=w890:bool)
            }
          }
        }
        n588 = flat-sequence {
          tunnel: w868 -> [_]
          frame #0 {
            n589 = local read "X Step Size"() -> (w879:dbl)
            n590 = local read "X Step Size"() -> (w875:dbl)
            n591 = Less?(x=w879, y=0.2) -> (x < y?=w876:bool)
            n592 = Less?(x=w875, y=0.4) -> (x < y?=w873:bool)
            n593 = Greater Or Equal?(x=w875, y=0.2) -> (x >= y?=w872:bool)
            n594 = Compound Arithmetic op=AND(w873, w872) -> (w871:bool)
            n595 = case shown="True" w876 {
              frame False {
              }
              frame True {
                n596 = local read "number of samples"() -> (w887:i32)
                n597 = Multiply(x=w887, y=0.15) -> (x*y=w884:dbl)
                n598 = Subtract(x=w887, y=w884) -> (x-y=w886:dbl)
                n599 = local write "number of samples"(w886) -> ()
              }
            }
            n600 = case shown="True" w871 {
              frame False {
              }
              frame True {
                n601 = local read "number of samples"() -> (w883:i32)
                n602 = Multiply(x=w883, y=0.075) -> (x*y=w881:dbl)
                n603 = Subtract(x=w883, y=w881) -> (x-y=w882:dbl)
                n604 = local write "number of samples"(w882) -> ()
              }
            }
          }
        }
      }
      frame "Line Scan" {
        n605 = local read "X=T,Y=F"() -> (w914:bool)
        n606 = local read "X Step Size"() -> (w910:dbl)
        n607 = case shown="True" w914 {
          tunnel: [w917 w918] -> w913
          frame False {
            n608 = local read "Y Step Size"() -> (w916:dbl)
            n609 = local read "Y Line Scan"() -> (w917:dbl[])
            n610 = local write "Y Step Size (in)"(w916) -> ()
          }
          frame True {
            n611 = local read "X Line Scan"() -> (w918:dbl[])
          }
        }
        n612 = local read "X Length"() -> (w912:dbl)
        n613 = local write "X Step Size (in)"(w910) -> ()
        n614 = while {
          tunnel: w914 -> [w932]
          shift-right: [w919] -> _
          shift-left: w913 -> [w925]
          tunnel: w912 -> [w922]
          tunnel: w910 -> [w921]
          tunnel: [w920] -> w911
          i -> [w931]
          stop <- w928 stop-if-true
          n615 = flat-sequence {
            tunnel: w932 -> [w938]
            tunnel: w931 -> [w935]
            tunnel: [w937] -> w930
            tunnel: [w936] -> w926
            tunnel: w925 -> [w936]
            tunnel: [w935] -> w923
            tunnel: w922 -> [w934]
            tunnel: w921 -> [w933]
            tunnel: w930 -> [w955]
            tunnel: [w954] -> w929
            tunnel: [w953] -> w927
            tunnel: w926 -> [w953]
            tunnel: [w952] -> w924
            tunnel: w923 -> [w952]
            tunnel: [w966] -> w928
            tunnel: w929 -> [w966]
            tunnel: w927 -> [w963]
            tunnel: [w962] -> w919
            tunnel: w924 -> [w961]
            tunnel: [w959] -> w920
            frame #0 {
              n616 = case shown="False" w938 {
                tunnel: w935 -> [w939 w947]
                tunnel: [w941 w948] -> w937
                tunnel: w934 -> [_ w946]
                tunnel: w933 -> [_ w945]
                frame False {
                  # "Had a +1"
                  n617 = local read "Y Step Size"() -> (w940:dbl)
                  n618 = local read "Y Length"() -> (w942:dbl)
                  n619 = property on="Move Y (in)" class="Bool (strict)"("Val(Sgnl)"=TRUE ("Value (Signaling)")) -> ()  [unwired: 2 in, 2 out]
                  n620 = Multiply(x=w939, y=w940) -> (x*y=w943:dbl)
                  n621 = Less Or Equal?(x=w942, y=w943) -> (x <= y?=w941:bool)
                }
                frame True {
                  n622 = property on="Move X (in)" class="Bool (strict)"("Val(Sgnl)"=TRUE ("Value (Signaling)")) -> ()  [unwired: 2 in, 2 out]
                  n623 = Multiply(x=w947, y=w945) -> (x*y=w949:dbl)
                  n624 = Less Or Equal?(x=w946, y=w949) -> (x <= y?=w948:bool)
                }
              }
            }
            frame #1 {
              n625 = while {
                tunnel: [w956] -> w951
                stop <- w958 stop-if-true
                n626 = local read "Abort"() -> (w956:bool)
                n627 = local read "Done Mov?"() -> (w957:bool)
                n628 = Or(x=w957, y=w956) -> (x .or. y?=w958:bool)
              }
              n629 = Or(x=w955, y=w951) -> (x .or. y?=w954:bool)
            }
            frame #2 {
              n630 = local read "number of samples"() -> (w964:i32)
              n631 = local read "task out"() -> (w965:refnum<k21>)
              n632 = local write "Done Mov?"(FALSE ("Done Moving?")) -> ()
              n633 = call "Measure Line Scan.vi"("number of samples per channel"=w964, "Iterator"=w961, "task/channels in"=w965, "Array in"=w963) -> ("task out"=w959:refnum<k21>, "Array out"=w962:dbl[])  [unwired: 4 in, 2 out]
            }
          }
          n634 = local write "Line Scan"(w919) -> ()
        }
        n635 = call <vilib>:"DAQmx Clear Task.vi"("task in"=w911) -> ()  [unwired: 14 in, 1 out]
      }
      frame "Flyover Linescan" {
        n636 = flat-sequence {
          tunnel: [w979] -> w971
          tunnel: [w984] -> w972
          tunnel: w971 -> [w985]
          tunnel: [w981] -> w969
          tunnel: w973 -> [w993]
          tunnel: w972 -> [w992]
          tunnel: "Measures/Pixel" -> [w990]
          tunnel: w969 -> [w989]
          tunnel: [w991] -> w968
          tunnel: [w988] -> w967
          tunnel: w968 -> [w1022]
          tunnel: w967 -> [w1020]
          frame #0 {
            n637 = local read "X Length"() -> (w978:dbl)
            n638 = local read "Y Length"() -> (w976:dbl)
            n639 = local write "Done Mov?"(FALSE ("Done Moving?")) -> ()
            n640 = local write "X Step Size (in)"(w978) -> ()
            n641 = local write "Y Step Size (in)"(w976) -> ()
            n642 = local read "task out"() -> (w979:refnum<k21>)
          }
          frame #1 {
            n643 = local read "X=T,Y=F"() -> (w983:bool)
            n644 = call <vilib>:"DAQmx Start Task.vi"("task/channels in"=w985) -> ("task out"=w984:refnum<k21>)  [unwired: 13 in, 1 out]
            n645 = case shown="False" w983 {
              frame False {
                n646 = property on="Move Y (in)" class="Bool (strict)"("Val(Sgnl)"=TRUE ("Value (Signaling)")) -> ()  [unwired: 2 in, 2 out]
              }
              frame True {
                n647 = property on="Move X (in)" class="Bool (strict)"("Val(Sgnl)"=TRUE ("Value (Signaling)")) -> ()  [unwired: 2 in, 2 out]
              }
            }
            n648 = Initialize Array(-inf, 1 ("dimension size")) -> (w981:dbl[])
          }
          frame #2 {
            n649 = while {
              tunnel: w993 -> [w1005]
              tunnel: w992 -> [w1004]
              tunnel: [w1003] -> w991
              tunnel: w990 -> [w999]
              shift-right: [w996] -> w988
              shift-left: w989 -> [w998]
              i -> [w997]
              stop <- w1000 stop-if-true
              n650 = while {
                tunnel: w1005 -> [w1010]
                tunnel: w1004 -> [w1013]
                tunnel: [w1012] -> w1003
                tunnel: w999 -> [w1007]
                tunnel: [w1006] -> w995 mode=indexing
                i -> [w1009]
                stop <- w1015 stop-if-true
                n651 = local read "Abort"() -> (w1014:bool)
                n652 = Greater?(x=w1009, y=w1007) -> (0:w1008:bool)
                n653 = Or(x=w1008, y=w1014) -> (x .or. y?=w1015:bool)
                n654 = call-poly <vilib>:"DAQmx Read.vi"("task/channels in"=w1013, "number of samples per channel"=w1010) -> ("task out"=w1012:refnum<k21>, "data"=w1011:dbl[])  [unwired: 11 in, 1 out]
                n655 = call-poly <vilib>:"Mean.vi"("X"=w1011) -> ("mean"=w1006:dbl)  [unwired: 1 out]
              }
              n656 = local read "Abort"() -> (w1002:bool)
              n657 = local read "Done Mov?"() -> (w1001:bool)
              n658 = Or(x=w1001, y=w1002) -> (x .or. y?=w1000:bool)
              n659 = call-poly <vilib>:"Mean.vi"("X"=w995) -> ("mean"=w994:dbl)  [unwired: 1 out]
              n660 = Insert Into Array(array=w998, index=w997, new element=w994) -> (w996:dbl[])
              n661 = local write "Line Scan"(w996) -> ()
            }
          }
          frame #3 {
            n662 = Array Size(array=w1020) -> (size(s)=w1019:i32)
            n663 = local read "X=T,Y=F"() -> (w1017:bool)
            n664 = call <vilib>:"DAQmx Stop Task.vi"("task/channels in"=w1022) -> ("task out"=w1023:refnum<k21>)  [unwired: 13 in, 1 out]
            n665 = local write "Done Mov?"(FALSE ("Done Mov?")) -> ()
            n666 = case shown="False" w1017 {
              tunnel: [w1024 w1025] -> w1016
              frame False {
                n667 = local read "Y Length"() -> (w1024:dbl)
              }
              frame True {
                n668 = local read "X Length"() -> (w1025:dbl)
              }
            }
            n669 = Divide(x=w1016, y=w1019) -> (x/y=w1018:dbl)
            n670 = call <vilib>:"DAQmx Clear Task.vi"("task in"=w1023) -> ()  [unwired: 14 in, 1 out]
            n671 = property on="Line Scan" class="WFGraph (strict)"("XScale.Multiplier"=w1018) -> ()  [unwired: 2 in, 2 out]
          }
        }
        n672 = local read "number of samples"() -> (w973:i32)
      }
      frame "Move to Origin" {
        n673 = local read "Acceleration"() -> (w1034:dbl)
        n674 = local read "Velocity"() -> (w1035:dbl)
        n675 = flat-sequence {
          tunnel: w1036 -> [_]
          tunnel: w1028 -> [w1052]
          tunnel: w1027 -> [w1051]
          frame #0 {
            n676 = while {
              stop <- w1050 stop-if-true
              n677 = local read "Done Mov?"() -> (w1050:bool)
              n678 = Wait (ms)(milliseconds to wait=u32 10) -> ()  [unwired: 1 out]
            }
          }
          frame #1 {
            n679 = local write "Done Mov?"(FALSE ("Done Mov?")) -> ()
            n680 = local write "Acceleration"(w1051) -> ()
            n681 = local write "Velocity"(w1052) -> ()
          }
          frame #2 {
            n682 = property on="Set Vel/Acc" class="Bool (strict)"("Val(Sgnl)"=TRUE ("Value (Signaling)")) -> ()  [unwired: 2 in, 2 out]
          }
          frame #3 {
            n683 = Wait (ms)(milliseconds to wait=u32 150) -> ()  [unwired: 1 out]
          }
        }
        n684 = flat-sequence {
          tunnel: w1035 -> [w1039]
          tunnel: w1034 -> [w1040]
          tunnel: [w1040] -> w1032
          tunnel: [w1039] -> w1030
          tunnel: [w1044] -> w1033
          tunnel: w1032 -> [w1044]
          tunnel: [w1043] -> w1031
          tunnel: w1030 -> [w1043]
          tunnel: [w1047] -> w1026
          tunnel: w1033 -> [w1047]
          tunnel: w1031 -> [w1046]
          tunnel: [w1046] -> w1029
          frame #0 {
            n685 = local write "Acceleration"(10.0 ("Acceleration")) -> ()
            n686 = local write "Velocity"(2.0 ("Velocity")) -> ()
          }
          frame #1 {
            n687 = property on="Set Vel/Acc" class="Bool (strict)"("Val(Sgnl)"=TRUE ("Value (Signaling)")) -> ()  [unwired: 2 in, 2 out]
          }
          frame #2 {
            n688 = Wait (ms)(milliseconds to wait=u32 150) -> ()  [unwired: 1 out]
          }
        }
        n689 = flat-sequence {
          tunnel: w1029 -> [w1057]
          tunnel: [w1057] -> w1028
          tunnel: [w1056] -> w1027
          tunnel: w1026 -> [w1056]
          tunnel: [w1073] -> w1036
          frame #0 {
            n690 = property on="Read Position" class="Bool (strict)"("Val(Sgnl)"=TRUE ("Value (Signaling)")) -> ()  [unwired: 2 in, 2 out]
            n691 = Wait (ms)(milliseconds to wait=u32 120) -> ()  [unwired: 1 out]
          }
          frame #1 {
            n692 = while {
              stop <- w1060 stop-if-true
              n693 = local read "Read Position"() -> (w1061:bool)
              n694 = Wait (ms)(milliseconds to wait=u32 10) -> ()  [unwired: 1 out]
              n695 = Not(x=w1061) -> (.not. x?=w1060:bool)
            }
          }
          frame #2 {
            n696 = local read "Y Origin"() -> (w1067:dbl)
            n697 = local read "X Origin"() -> (w1064:dbl)
            n698 = local read "Y Pos"() -> (w1066:dbl)
            n699 = local read "X Pos"() -> (w1063:dbl)
            n700 = Subtract(x=w1064, y=w1063) -> (x-y=w1065:dbl)
            n701 = Subtract(x=w1067, y=w1066) -> (x-y=w1068:dbl)
            n702 = local write "X Step Size (in)"(w1065) -> ()
            n703 = local write "Y Step Size (in)"(w1068) -> ()
          }
          frame #3 {
            n704 = local write "Done Mov?"(FALSE ("Done Mov?")) -> ()
          }
          frame #4 {
            n705 = property on="Move X (in)" class="Bool (strict)"("Val(Sgnl)"=TRUE ("Value (Signaling)")) -> ()  [unwired: 2 in, 2 out]
          }
          frame #5 {
            n706 = while {
              stop <- w1071 stop-if-true
              n707 = local read "Done Mov?"() -> (w1071:bool)
            }
          }
          frame #6 {
            n708 = local write "Done Mov?"(FALSE ("Done Mov?")) -> ()
          }
          frame #7 {
            n709 = property on="Move Y (in)" class="Bool (strict)"("Val(Sgnl)"=TRUE ("Value (Signaling)")) -> (error out=w1073:errorcluster)  [unwired: 2 in, 1 out]
          }
        }
      }
      frame "Move to Saved Position" {
        n710 = flat-sequence {
          tunnel: [w1095] -> w1075
          frame #0 {
            n711 = property on="Read Position" class="Bool (strict)"("Val(Sgnl)"=TRUE ("Value (Signaling)")) -> ()  [unwired: 2 in, 2 out]
            n712 = Wait (ms)(milliseconds to wait=u32 120) -> ()  [unwired: 1 out]
          }
          frame #1 {
            n713 = while {
              stop <- w1083 stop-if-true
              n714 = local read "Read Position"() -> (w1084:bool)
              n715 = Wait (ms)(milliseconds to wait=u32 10) -> ()  [unwired: 1 out]
              n716 = Not(x=w1084) -> (.not. x?=w1083:bool)
            }
          }
          frame #2 {
            n717 = local read "X Pos 1"() -> (w1090:dbl)
            n718 = local read "Y Pos 1"() -> (w1088:dbl)
            n719 = local read "X Pos"() -> (w1091:dbl)
            n720 = local read "Y Pos"() -> (w1087:dbl)
            n721 = Subtract(x=w1090, y=w1091) -> (x-y=w1089:dbl)
            n722 = Subtract(x=w1088, y=w1087) -> (x-y=w1086:dbl)
            n723 = local write "Y Step Size (in)"(w1086) -> ()
            n724 = local write "X Step Size (in)"(w1089) -> ()
          }
          frame #3 {
            n725 = local write "Done Mov?"(FALSE ("Done Mov?")) -> ()
            n726 = property on="Move X (in)" class="Bool (strict)"("Val(Sgnl)"=TRUE ("Value (Signaling)")) -> ()  [unwired: 2 in, 2 out]
          }
          frame #4 {
            n727 = while {
              stop <- w1094 stop-if-true
              n728 = local read "Done Mov?"() -> (w1094:bool)
            }
          }
          frame #5 {
            n729 = local write "Done Mov?"(FALSE ("Done Mov?")) -> ()
            n730 = property on="Move Y (in)" class="Bool (strict)"("Val(Sgnl)"=TRUE ("Value (Signaling)")) -> (error out=w1095:errorcluster)  [unwired: 2 in, 1 out]
          }
        }
        n731 = flat-sequence {
          tunnel: w1075 -> [_]
          frame #0 {
            n732 = while {
              stop <- w1079 stop-if-true
              n733 = local read "Done Mov?"() -> (w1079:bool)
              n734 = Wait (ms)(milliseconds to wait=u32 10) -> ()  [unwired: 1 out]
            }
          }
          frame #1 {
            n735 = local write "Done Mov?"(FALSE ("Done Mov?")) -> ()
          }
        }
      }
      frame "Move to Cursor" {
        n736 = flat-sequence {
          tunnel: w1100 -> [_]
          tunnel: [w1113] -> w1104
          tunnel: w1104 -> [w1123]
          tunnel: [w1124] -> w1098
          tunnel: [w1126] -> w1099
          tunnel: w1098 -> [w1126]
          frame #0 {
            n737 = while {
              stop <- w1111 stop-if-true
              n738 = local read "Read Position"() -> (w1112:bool)
              n739 = Not(x=w1112) -> (.not. x?=w1111:bool)
              n740 = Wait (ms)(milliseconds to wait=u32 10) -> ()  [unwired: 1 out]
            }
          }
          frame #1 {
            n741 = property on="Graph" class="IntGraph (strict)"("Active Cursor"=u32 0) -> (error out=w1114:errorcluster)  [unwired: 2 in, 1 out]
            n742 = property on="Graph" class="IntGraph (strict)"(error in=w1114) -> ("Cursor.Cursor Position"=w1113:T3)  [unwired: 1 in, 2 out]
          }
          frame #2 {
            n743 = Unbundle By Name(w1123) -> ("Cursor X"=w1122:dbl, "Cursor Y"=w1117:dbl)
            n744 = local read "X Pos"() -> (w1121:dbl)
            n745 = local read "Y Pos"() -> (w1120:dbl)
            n746 = Subtract(x=w1122, y=w1121) -> (x-y=w1119:dbl)
            n747 = Subtract(x=w1117, y=w1120) -> (x-y=w1118:dbl)
            n748 = local write "X Step Size (in)"(w1119) -> ()
            n749 = local write "Y Step Size (in)"(w1118) -> ()
            n750 = local write "Done Mov?"(FALSE ("Done Mov?")) -> ()
          }
          frame #3 {
            n751 = property on="Move Y (in)" class="Bool (strict)"("Val(Sgnl)"=TRUE) -> (error out=w1124:errorcluster)  [unwired: 2 in, 1 out]
          }
          frame #4 {
            n752 = while {
              stop <- w1128 stop-if-true
              n753 = local read "Done Mov?"() -> (w1128:bool)
              n754 = Wait (ms)(milliseconds to wait=u32 10 ("millisecond timer value")) -> ()  [unwired: 1 out]
            }
          }
        }
        n755 = property on="Read Position" class="Bool (strict)"("Val(Sgnl)"=TRUE) -> (error out=w1100:errorcluster)  [unwired: 2 in, 1 out]
        n756 = flat-sequence {
          tunnel: w1099 -> [_]
          frame #0 {
            n757 = local write "Done Mov?"(FALSE ("Done Mov?")) -> ()
            n758 = property on="Move X (in)" class="Bool (strict)"("Val(Sgnl)"=TRUE) -> ()  [unwired: 2 in, 2 out]
          }
          frame #1 {
            n759 = while {
              stop <- w1107 stop-if-true
              n760 = local read "Done Mov?"() -> (w1107:bool)
              n761 = Wait (ms)(milliseconds to wait=u32 10 ("millisecond timer value")) -> ()  [unwired: 1 out]
            }
          }
          frame #2 {
            n762 = local write "Done Mov?"(FALSE ("Done Mov?")) -> ()
          }
        }
      }
      frame "Move to Cursor 2" {
        n763 = flat-sequence {
          tunnel: w1131 -> [_]
          tunnel: [w1144] -> w1135
          tunnel: w1135 -> [w1154]
          tunnel: [w1155] -> w1129
          tunnel: [w1157] -> w1130
          tunnel: w1129 -> [w1157]
          frame #0 {
            n764 = while {
              stop <- w1142 stop-if-true
              n765 = local read "Read Position"() -> (w1143:bool)
              n766 = Not(x=w1143) -> (.not. x?=w1142:bool)
              n767 = Wait (ms)(milliseconds to wait=u32 10) -> ()  [unwired: 1 out]
            }
          }
          frame #1 {
            n768 = property on="Graph 2" class="IntGraph (strict)"("Active Cursor"=u32 0) -> (error out=w1146:errorcluster)  [unwired: 2 in, 1 out]
            n769 = property on="Graph 2" class="IntGraph (strict)"(error in=w1146) -> ("Cursor.Cursor Position"=w1144:T3)  [unwired: 1 in, 2 out]
          }
          frame #2 {
            n770 = Unbundle By Name(w1154) -> ("Cursor X"=w1153:dbl, "Cursor Y"=w1148:dbl)
            n771 = local read "X Pos"() -> (w1152:dbl)
            n772 = local read "Y Pos"() -> (w1151:dbl)
            n773 = Subtract(x=w1153, y=w1152) -> (x-y=w1150:dbl)
            n774 = Subtract(x=w1148, y=w1151) -> (x-y=w1149:dbl)
            n775 = local write "X Step Size (in)"(w1150) -> ()
            n776 = local write "Y Step Size (in)"(w1149) -> ()
            n777 = local write "Done Mov?"(FALSE ("Done Mov?")) -> ()
          }
          frame #3 {
            n778 = property on="Move Y (in)" class="Bool (strict)"("Val(Sgnl)"=TRUE) -> (error out=w1155:errorcluster)  [unwired: 2 in, 1 out]
          }
          frame #4 {
            n779 = while {
              stop <- w1159 stop-if-true
              n780 = local read "Done Mov?"() -> (w1159:bool)
              n781 = Wait (ms)(milliseconds to wait=u32 10 ("millisecond timer value")) -> ()  [unwired: 1 out]
            }
          }
        }
        n782 = property on="Read Position" class="Bool (strict)"("Val(Sgnl)"=TRUE) -> (error out=w1131:errorcluster)  [unwired: 2 in, 1 out]
        n783 = flat-sequence {
          tunnel: w1130 -> [_]
          frame #0 {
            n784 = local write "Done Mov?"(FALSE ("Done Mov?")) -> ()
            n785 = property on="Move X (in)" class="Bool (strict)"("Val(Sgnl)"=TRUE) -> ()  [unwired: 2 in, 2 out]
          }
          frame #1 {
            n786 = while {
              stop <- w1138 stop-if-true
              n787 = local read "Done Mov?"() -> (w1138:bool)
              n788 = Wait (ms)(milliseconds to wait=u32 10 ("millisecond timer value")) -> ()  [unwired: 1 out]
            }
          }
          frame #2 {
            n789 = local write "Done Mov?"(FALSE ("Done Mov?")) -> ()
          }
        }
      }
      frame "Move to" {
        n790 = flat-sequence {
          frame #0 {
            n791 = property on="Read Position" class="Bool (strict)"("Val(Sgnl)"=TRUE ("Value (Signaling)")) -> ()  [unwired: 2 in, 2 out]
          }
          frame #1 {
            n792 = while {
              stop <- w1163 stop-if-true
              n793 = local read "Read Position"() -> (w1165:bool)
              n794 = Wait (ms)(milliseconds to wait=u32 10) -> ()  [unwired: 1 out]
              n795 = Not(x=w1165) -> (.not. x?=w1163:bool)
            }
          }
          frame #2 {
            n796 = local read "X=T,Y=F"() -> (w1167:bool)
            n797 = case shown="False" w1167 {
              tunnel: [w1169 w1175] -> w1166
              frame False {
                n798 = flat-sequence {
                  tunnel: [w1173] -> w1169
                  frame #0 {
                    n799 = local read "Y Pos"() -> (w1171:dbl)
                    n800 = Subtract(x="Y Move", y=w1171) -> (x-y=w1170:dbl)
                    n801 = local write "Y Step Size (in)"(w1170) -> ()
                  }
                  frame #1 {
                    n802 = property on="Move Y (in)" class="Bool (strict)"("Val(Sgnl)"=TRUE ("Value (Signaling)")) -> (error out=w1173:errorcluster)  [unwired: 2 in, 1 out]
                  }
                }
              }
              frame True {
                n803 = flat-sequence {
                  tunnel: [w1179] -> w1175
                  frame #0 {
                    n804 = local read "X Pos"() -> (w1178:dbl)
                    n805 = Subtract(x="X Move", y=w1178) -> (x-y=w1176:dbl)
                    n806 = local write "X Step Size (in)"(w1176) -> ()
                  }
                  frame #1 {
                    n807 = property on="Move X (in)" class="Bool (strict)"("Val(Sgnl)"=TRUE ("Value (Signaling)")) -> (error out=w1179:errorcluster)  [unwired: 2 in, 1 out]
                  }
                }
              }
            }
            n808 = while {
              tunnel: w1166 -> [_]
              stop <- w1168 stop-if-true
              n809 = local read "Done Mov?"() -> (w1168:bool)
            }
          }
        }
      }
      frame "Update Vel/Acc" {
        n810 = flat-sequence {
          frame #0 {
            n811 = property on="Set Vel/Acc" class="Bool (strict)"("Val(Sgnl)"=TRUE ("Value (Signaling)")) -> ()  [unwired: 2 in, 2 out]
          }
          frame #1 {
            n812 = Wait (ms)(milliseconds to wait=u32 50) -> ()  [unwired: 1 out]
          }
        }
      }
      frame "Convert" {
        w1191 = 0 ("index")
        w1192 = 0 ("index")
        w1220 = path "C:/Users/mnopl/OneDrive/Documents/PhiThetaScanning/GridDataScript.py" ("module path")
        n813 = local read "(X,Y)"() -> (w1197:cluster{dbl, dbl}[][])
        n814 = local read "Scan Type"() -> (w1189:string)
        n815 = local read "array of values"() -> (w1195:dbl[][])
        n816 = disable-structure shown="Enabled" {
          disable-tunnel: [w1273 w1291] -> w1204
          disable-tunnel: w1195 -> [w1267 w1291]
          frame Enabled {
            n817 = Array Size(array=w1267) -> (size(s)=w1270:i32[])
            n818 = Index Array(array=w1270, index=1) -> (element=w1268:i32)
            n819 = Index Array(array=w1270, index=0) -> (element=w1269:i32)
            n820 = for {
              N: w1269 -> [_]
              shift-right: [w1275] -> w1273
              shift-left: w1267 -> [w1276]
              tunnel: w1268 -> [w1274]
              i -> [w1277]
              n821 = for {
                N: w1274 -> [_]
                tunnel: w1277 -> [w1280]
                shift-right: [w1278] -> w1275
                shift-left: w1276 -> [w1281]
                i -> [w1279]
                n822 = Index Array(array=w1281, index (row)=w1279, index (col)=w1280) -> (element=w1284:dbl)
                n823 = Equal?(x=-inf, y=w1284) -> (x = y?=w1282:bool)
                n824 = case shown="True" w1282 {
                  tunnel: w1281 -> [w1285 w1290]
                  tunnel: w1280 -> [_ w1289]
                  tunnel: w1279 -> [_ w1288]
                  tunnel: [w1285 w1286] -> w1278
                  frame False {
                  }
                  frame True {
                    n825 = Replace Array Subset(array=w1290, new element=-100.0 ("new element/subarray"), index (row)=w1288, index (col)=w1289) -> (w1286:dbl[][])
                  }
                }
              }
            }
          }
          frame Disabled {
          }
        }
        n826 = Array Size(array=w1204) -> (size(s)=w1199:i32[])
        n827 = Equal?(x=w1189, y="Flyover Scan") -> (x = y?=w1187:bool)
        n828 = case shown="True" w1187 {
          tunnel: w1199 -> [_ w1250]
          tunnel: w1197 -> [w1246 _]
          tunnel: [w1246 w1247] -> w1196
          frame False {
          }
          frame True {
            n829 = Index Array(array=w1250, index=0) -> (element=w1252:i32)
            n830 = Index Array(array=w1250, index=1) -> (element=w1248:i32)
            n831 = for {
              N: w1252 -> [_]
              tunnel: w1248 -> [w1255]
              tunnel: [w1254] -> w1247 mode=indexing
              i -> [w1253]
              n832 = for {
                N: w1255 -> [_]
                tunnel: [w1266] -> w1254 mode=indexing
                tunnel: w1253 -> [w1265]
                i -> [w1264]
                n833 = local read "X Step Size"() -> (w1262:dbl)
                n834 = local read "Y Step Size"() -> (w1263:dbl)
                n835 = Multiply(x=w1263, y=w1265) -> (x*y=w1257:dbl)
                n836 = property on="Graph" class="IntGraph (strict)"() -> ("XScale.Offset"=w1260:dbl)  [unwired: 2 in, 2 out]
                n837 = Multiply(x=w1262, y=w1264) -> (x*y=w1259:dbl)
                n838 = property on="Graph" class="IntGraph (strict)"() -> ("YScale.Offset"=w1256:dbl)  [unwired: 2 in, 2 out]
                n839 = Add(x=w1260, y=w1259) -> (x+y=w1261:dbl)
                n840 = Add(x=w1257, y=w1256) -> (x+y=w1258:dbl)
                n841 = Bundle(w1261, w1258) -> (w1266:cluster{dbl, dbl})  [unwired: 1 in]
              }
            }
          }
        }
        n842 = disable-structure shown="Enabled" {
          disable-tunnel: [w1244 w1245] -> w1200
          disable-tunnel: w1196 -> [w1243 w1245]
          frame Disabled {
            n843 = Transpose 2D Array(2D array=w1243) -> (transposed array=w1244:cluster{dbl, dbl}[][])
          }
          frame Enabled {
          }
        }
        n844 = Array Size(array=w1200) -> (size(s)=w1227:i32[])
        n845 = Index Array(array=w1227, index=0) -> (element=w1190:i32)
        n846 = Index Array(array=w1227, index=1) -> (element=w1223:i32)
        n847 = for {
          N: w1190 -> [_]
          tunnel: w1200 -> [w1299]
          tunnel: [w1297] -> w1202 mode=indexing
          tunnel: w1223 -> [w1296]
          i -> [w1298]
          n848 = for {
            N: w1296 -> [_]
            tunnel: w1299 -> [w1310]
            tunnel: w1298 -> [w1308]
            tunnel: [w1302] -> w1297 mode=indexing
            i -> [w1309]
            n849 = Index Array(array=w1310, index (row)=w1308, index (col)=w1309) -> (element=w1305:cluster{dbl, dbl})
            n850 = Unbundle(w1305) -> (w1304:dbl, w1303:dbl)
            n851 = Subtract(x=w1304, y="X Center") -> (x-y=w1307:dbl)
            n852 = Subtract(x=w1303, y="Y Center") -> (x-y=w1306:dbl)
            n853 = Bundle(w1307, w1306) -> (w1302:cluster{dbl, dbl})  [unwired: 1 in]
          }
        }
        n854 = Array Subset(array=w1204, index (row)=w1191, length (row)=w1190, index (col)=w1191, length (col)=w1223) -> (w1222:dbl[][])
        n855 = Index Array(array=w1199, index=1) -> (element=w1193:i32)
        n856 = Index Array(array=w1199, index=0) -> (element=w1224:i32)
        n857 = local write "(X,Y)"(w1196) -> ()
        n858 = Array Subset(array=w1202, index (row)=w1192, length (row)=w1224, index (col)=w1192, length (col)=w1193) -> (w1198:cluster{dbl, dbl}[][])
        n859 = node(w1203, w1220, "grid" ("function name"), w1222, w1198, w1222, "Grid points") -> (w1221:refnum<k35>, w1214:errorcluster, w1186:dbl[][])  [unwired: 4 in, 2 out]
        n860 = disable-structure shown="Enabled" {
          disable-tunnel: w1186 -> [w1241 w1242]
          disable-tunnel: [w1240 w1242] -> w1185
          frame Enabled {
            n861 = Transpose 2D Array(2D array=w1241) -> (transposed array=w1240:dbl[][])
          }
          frame Disabled {
          }
        }
        n862 = Initialize Array(0.0 ("element"), 4 ("dimension size")) -> (w1216:dbl[])
        n863 = flat-sequence {
          tunnel: w1185 -> [w1293]
          tunnel: [w1292] -> w1201
          tunnel: w1201 -> [w1294]
          frame #0 {
            n864 = local write "Phi Theta Data"(w1293) -> ()
            n865 = Array Max & Min(array=w1293) -> (max value=w1292:dbl)  [unwired: 3 out]
          }
          frame #1 {
            n866 = property on="Graph" class="IntGraph (strict)"() -> ("ZScale.Minimum"=w1295:dbl)  [unwired: 2 in, 2 out]
            n867 = property on="Phi Theta Data" class="IntGraph (strict)"("ZScale.Maximum"=w1294, "ZScale.Minimum"=w1295) -> ()  [unwired: 2 in, 2 out]
          }
        }
        n868 = node(w1221, w1220, "OffsetAndMult" ("function name"), w1214, w1216, "Grid points") -> (w1215:dbl[])  [unwired: 1 in, 4 out]
        n869 = Index Array(array=w1215, index=0) -> (element=w1209:dbl)
        n870 = Index Array(array=w1215, index=1) -> (element=w1208:dbl)
        n871 = Index Array(array=w1215, index=2) -> (element=w1207:dbl)
        n872 = Index Array(array=w1215, index=3) -> (element=w1206:dbl)
        n873 = disable-structure shown="Enabled" {
          disable-tunnel: w1209 -> [w1235 w1239]
          disable-tunnel: w1208 -> [w1234 w1238]
          disable-tunnel: w1207 -> [w1233 w1237]
          disable-tunnel: w1206 -> [w1232 w1236]
          frame Disabled {
            n874 = property on="Phi Theta Data" class="IntGraph (strict)"("XScale.Multiplier"=w1234, "XScale.Offset"=w1235) -> ()  [unwired: 2 in, 2 out]
            n875 = property on="Phi Theta Data" class="IntGraph (strict)"("YScale.Multiplier"=w1232, "YScale.Offset"=w1233) -> ()  [unwired: 2 in, 2 out]
          }
          frame Enabled {
            n876 = property on="Phi Theta Data" class="IntGraph (strict)"("YScale.Multiplier"=w1238, "YScale.Offset"=w1239) -> ()  [unwired: 2 in, 2 out]
            n877 = property on="Phi Theta Data" class="IntGraph (strict)"("XScale.Multiplier"=w1236, "XScale.Offset"=w1237) -> ()  [unwired: 2 in, 2 out]
          }
        }
      }
      frame "Save Position" {
        n878 = flat-sequence {
          frame #0 {
            n879 = property on="Read Position" class="Bool (strict)"("Val(Sgnl)"=TRUE ("Value (Signaling)")) -> ()  [unwired: 2 in, 2 out]
          }
          frame #1 {
            n880 = while {
              stop <- w1315 stop-if-true
              n881 = local read "Read Position"() -> (w1316:bool)
              n882 = Wait (ms)(milliseconds to wait=u32 10) -> ()  [unwired: 1 out]
              n883 = Not(x=w1316) -> (.not. x?=w1315:bool)
            }
          }
          frame #2 {
            n884 = local read "X Pos"() -> (→"X Pos 1":dbl)
            n885 = local read "Y Pos"() -> (→"Y Pos 1":dbl)
          }
        }
      }
      frame "Save Image" {
        n886 = property on="Graph" class="IntGraph (strict)"("Active Cursor"=u32 0) -> (error out=w1330:errorcluster)  [unwired: 2 in, 1 out]
        n887 = property on="Graph" class="IntGraph (strict)"(error in=w1330, "Cursor.Visible"=FALSE) -> (error out=w1324:errorcluster)  [unwired: 1 in, 1 out]
        n888 = property on="Graph" class="IntGraph (strict)"(error in=w1324, "Cursor Palette Vis"=FALSE ("Cursor Legend Visible")) -> (error out=w1319:errorcluster)  [unwired: 1 in, 1 out]
        n889 = invoke on="Graph" class="IntGraph (strict)" method="Get Image"(error in=w1319, "image depth"=24 ("Image Depth")) -> (error out=w1326:errorcluster, "image data"=w1327:T4)  [unwired: 4 in, 4 out]
        n890 = call <vilib>:"Write PNG File.vi"("error in (no error)"=w1326, "image data"=w1327) -> ("error out"=w1323:errorcluster)  [unwired: 8 in, 1 out]
        n891 = property on="Graph" class="IntGraph (strict)"(error in=w1323, "Cursor.Visible"=TRUE) -> (error out=w1322:errorcluster)  [unwired: 1 in, 1 out]
        n892 = property on="Graph" class="IntGraph (strict)"(error in=w1322, "Cursor Palette Vis"=TRUE ("Cursor.Visible")) -> ()  [unwired: 1 in, 2 out]
      }
      frame "Save Image 2" {
        n893 = property on="Graph 2" class="IntGraph (strict)"("Active Cursor"=u32 0) -> (error out=w1344:errorcluster)  [unwired: 2 in, 1 out]
        n894 = property on="Graph 2" class="IntGraph (strict)"(error in=w1344, "Cursor.Visible"=FALSE) -> (error out=w1345:errorcluster)  [unwired: 1 in, 1 out]
        n895 = property on="Graph 2" class="IntGraph (strict)"(error in=w1345, "Cursor Palette Vis"=FALSE ("Cursor Legend Visible")) -> (error out=w1346:errorcluster)  [unwired: 1 in, 1 out]
        n896 = invoke on="Graph 2" class="IntGraph (strict)" method="Get Image"(error in=w1346, "image depth"=24 ("Image Depth")) -> (error out=w1339:errorcluster, "image data"=w1338:T4)  [unwired: 4 in, 4 out]
        n897 = call <vilib>:"Write PNG File.vi"("error in (no error)"=w1339, "image data"=w1338) -> ("error out"=w1337:errorcluster)  [unwired: 8 in, 1 out]
        n898 = property on="Graph 2" class="IntGraph (strict)"(error in=w1337, "Cursor.Visible"=TRUE) -> (error out=w1336:errorcluster)  [unwired: 1 in, 1 out]
        n899 = property on="Graph 2" class="IntGraph (strict)"(error in=w1336, "Cursor Palette Vis"=TRUE ("Cursor Legend Visible")) -> ()  [unwired: 1 in, 2 out]
      }
      frame "Save Data" {
        w1360 = 0 ("index")
        w1371 = 0
        n900 = local read "(X,Y)"() -> (w1358:cluster{dbl, dbl}[][])
        n901 = Array Size(array=w1358) -> (size(s)=w1353:i32[])
        n902 = Index Array(array=w1353, index=0) -> (element=w1356:i32)
        n903 = Index Array(array=w1353, index=1) -> (element=w1355:i32)
        n904 = for {
          N: w1356 -> [_]
          tunnel: w1358 -> [w1391]
          tunnel: [w1389] -> w1359 mode=indexing
          tunnel: w1355 -> [w1388]
          i -> [w1390]
          n905 = for {
            N: w1388 -> [_]
            tunnel: w1391 -> [w1402]
            tunnel: w1390 -> [w1400]
            tunnel: [w1394] -> w1389 mode=indexing
            i -> [w1401]
            n906 = Index Array(array=w1402, index (row)=w1400, index (col)=w1401) -> (element=w1397:cluster{dbl, dbl})
            n907 = local read "X Center"() -> (w1393:dbl)
            n908 = local read "Y Center"() -> (w1392:dbl)
            n909 = Unbundle(w1397) -> (w1396:dbl, w1395:dbl)
            n910 = Subtract(x=w1395, y=w1392) -> (x-y=w1398:dbl)
            n911 = Subtract(x=w1396, y=w1393) -> (x-y=w1399:dbl)
            n912 = Bundle(w1399, w1398) -> (w1394:cluster{dbl, dbl})  [unwired: 1 in]
          }
        }
        n913 = local read "array of values"() -> (w1372:dbl[][])
        n914 = Array Size(array=w1359) -> (size(s)=w1368:i32[])
        n915 = Index Array(array=w1368, index=0) -> (element=w1369:i32)
        n916 = Index Array(array=w1368, index=1) -> (element=w1366:i32)
        n917 = Array Size(array=w1372) -> (size(s)=w1365:i32[])
        n918 = Array Subset(array=w1372, index (row)=w1371, length (row)=w1369, index (col)=w1371, length (col)=w1366) -> (w1351:dbl[][])
        n919 = Index Array(array=w1365, index=0) -> (element=w1361:i32)
        n920 = Index Array(array=w1365, index=1) -> (element=w1362:i32)
        n921 = Array Subset(array=w1359, index (row)=w1360, length (row)=w1361, index (col)=w1360, length (col)=w1362) -> (w1350:cluster{dbl, dbl}[][])
        n922 = node(w1378, path "C:/Users/mnopl/OneDrive/Documents/PhiThetaScanning/SaveDataToTextFiles.py" ("module path"), "savedata" ("function name"), w1351, w1350, w1351, "Name of File") -> (w1349:refnum<k35>, w1373:dbl[][])  [unwired: 4 in, 3 out]
        n923 = disable-structure shown="Enabled" {
          disable-tunnel: w1351 -> [w1382 _]
          disable-tunnel: w1350 -> [w1381 _]
          disable-tunnel: w1349 -> [w1379 _]
          frame Disabled {
            n924 = local read "Grid points"() -> (w1385:dbl)
            n925 = node(w1379, path "C:/Users/mnopl/OneDrive/Documents/PhiThetaScanning/GridDataScript.py" ("module path"), "grid" ("function name"), w1382, w1381, w1382, w1385) -> (w1380:dbl[][])  [unwired: 4 in, 4 out]
            n926 = local write "Phi Theta Data"(w1380) -> ()
          }
          frame Enabled {
          }
        }
        n927 = flat-sequence {
          tunnel: w1373 -> [w1387]
          frame #0 {
            n928 = local write "Name of File"(" " ("Name of File")) -> ()
            "return value" <- w1387
          }
        }
      }
      frame "Save Phi/Theta" {
        n929 = property on="Phi Theta Data" class="IntGraph (strict)"("Active Cursor"=u32 0) -> (error out=w1413:errorcluster)  [unwired: 2 in, 1 out]
        n930 = property on="Phi Theta Data" class="IntGraph (strict)"(error in=w1413, "Cursor.Visible"=FALSE) -> (error out=w1411:errorcluster)  [unwired: 1 in, 1 out]
        n931 = property on="Phi Theta Data" class="IntGraph (strict)"(error in=w1411, "Cursor Palette Vis"=FALSE ("Cursor Legend Visible")) -> (error out=w1409:errorcluster)  [unwired: 1 in, 1 out]
        n932 = invoke on="Phi Theta Data" class="IntGraph (strict)" method="Get Image"(error in=w1409, "image depth"=24 ("Image Depth")) -> ("image data"=w1408:T4)  [unwired: 4 in, 5 out]
        n933 = call <vilib>:"Write PNG File.vi"("image data"=w1408) -> ("error out"=w1407:errorcluster)  [unwired: 9 in, 1 out]
        n934 = property on="Phi Theta Data" class="IntGraph (strict)"(error in=w1407, "Cursor.Visible"=TRUE) -> (error out=w1406:errorcluster)  [unwired: 1 in, 1 out]
        n935 = property on="Phi Theta Data" class="IntGraph (strict)"(error in=w1406, "Cursor Palette Vis"=TRUE ("Cursor Legend Visible")) -> ()  [unwired: 1 in, 2 out]
      }
      frame "Save Line graph" {
        n936 = property on="Line Scan" class="WFGraph (strict)"("Active Cursor"=u32 0) -> (error out=w1423:errorcluster)  [unwired: 2 in, 1 out]
        n937 = property on="Line Scan" class="WFGraph (strict)"(error in=w1423, "Cursor.Visible"=FALSE) -> (error out=w1424:errorcluster)  [unwired: 1 in, 1 out]
        n938 = property on="Line Scan" class="WFGraph (strict)"(error in=w1424, "Cursor Palette Vis"=FALSE ("Cursor Legend Visible")) -> (error out=w1425:errorcluster)  [unwired: 1 in, 1 out]
        n939 = invoke on="Line Scan" class="WFGraph (strict)" method="Get Image"(error in=w1425, "image depth"=24 ("Image Depth")) -> (error out=w1427:errorcluster, "image data"=w1426:T4)  [unwired: 4 in, 4 out]
        n940 = call <vilib>:"Write PNG File.vi"("error in (no error)"=w1427, "image data"=w1426) -> ("error out"=w1428:errorcluster)  [unwired: 8 in, 1 out]
        n941 = property on="Line Scan" class="WFGraph (strict)"(error in=w1428, "Cursor.Visible"=TRUE) -> (error out=w1429:errorcluster)  [unwired: 1 in, 1 out]
        n942 = property on="Line Scan" class="WFGraph (strict)"(error in=w1429, "Cursor Palette Vis"=TRUE ("Cursor Legend Visible")) -> ()  [unwired: 1 in, 2 out]
      }
      frame "Save Line graph 2" {
        n943 = property on="Line Scan 2" class="WFGraph (strict)"("Active Cursor"=u32 0) -> (error out=w1442:errorcluster)  [unwired: 2 in, 1 out]
        n944 = property on="Line Scan 2" class="WFGraph (strict)"(error in=w1442, "Cursor.Visible"=FALSE) -> (error out=w1441:errorcluster)  [unwired: 1 in, 1 out]
        n945 = property on="Line Scan 2" class="WFGraph (strict)"(error in=w1441, "Cursor Palette Vis"=FALSE ("Cursor Legend Visible")) -> (error out=w1438:errorcluster)  [unwired: 1 in, 1 out]
        n946 = invoke on="Line Scan 2" class="WFGraph (strict)" method="Get Image"(error in=w1438) -> (error out=w1437:errorcluster, "image data"=w1436:T4)  [unwired: 5 in, 4 out]
        n947 = call <vilib>:"Write PNG File.vi"("error in (no error)"=w1437, "image data"=w1436) -> ("error out"=w1435:errorcluster)  [unwired: 8 in, 1 out]
        n948 = property on="Line Scan 2" class="WFGraph (strict)"(error in=w1435, "Cursor.Visible"=TRUE) -> (error out=w1433:errorcluster)  [unwired: 1 in, 1 out]
        n949 = property on="Line Scan 2" class="WFGraph (strict)"(error in=w1433, "Cursor Palette Vis"=TRUE ("Cursor Legend Visible")) -> ()  [unwired: 1 in, 2 out]
      }
      frame "Stop" {
      }
    }
  }
  n950 = while {
    shift-right: [w1448] -> _
    shift-left: "Idle" -> [w1450]
    tunnel: w18 -> [_]
    tunnel: w17 -> [_]
    stop <- w1449 stop-if-true
    n951 = case shown="\"Moving\"" w1450 {
      tunnel: [w1452 "Stop" "Idle" "Idle"] -> w1448
      tunnel: [FALSE TRUE FALSE FALSE] -> w1449
      frame "Idle", Default {
        n952 = flat-sequence {
          frame #0 {
            w1453 = FALSE
            n953 = local write "Move X (in)"(w1453) -> ()
            n954 = local write "Move Y (in)"(w1453) -> ()
            n955 = local write "Take Single Measurement"(w1453) -> ()
            n956 = local write "Moving?"(w1453) -> ()
            n957 = local write "Move X"(w1453) -> ()
            n958 = local write "Move Y"(w1453) -> ()
          }
        }
        n959 = event shown="[5] \"Move Y (in)\": Value Change" {
          selector: _ -> [_ _ _ _ _ _ _]
          dyn-events: _ -> [_ _ _ _ _ _ _]
          timeout: _ -> [_ _ _ _ w1461 _ _]
          tunnel: ["Wait" "Stop" "Moving" "Moving" "Moving" "Moving" "Idle"] -> w1452
          tunnel: [_ _ _ _ w1461 _ _] -> _
          event Timeout {
            n960 = event-data() -> ()  [unwired: 1 in, 3 out]
          }
          event "Stop": Value Change {
            n961 = event-data() -> ()  [unwired: 1 in, 6 out]
          }
          event "Move X (in)": Value Change {
            n962 = event-data() -> ()  [unwired: 1 in, 6 out]
            n963 = local write "X=T,Y=F"(TRUE) -> ()
          }
          event "Move X": Value Change {
            n964 = event-data() -> ()  [unwired: 1 in, 6 out]
            n965 = local write "X Step Size (in)"("X Step Size") -> ()
            n966 = local write "X=T,Y=F"(TRUE ("X=T,Y=F")) -> ()
          }
          event "Move Y": Value Change {
            n967 = event-data() -> ()  [unwired: 1 in, 6 out]
            n968 = local write "X=T,Y=F"(FALSE ("X=T,Y=F")) -> ()
            n969 = local write "Y Step Size (in)"("Y Step Size") -> ()
          }
          event "Move Y (in)": Value Change {
            n970 = event-data() -> ()  [unwired: 1 in, 6 out]
            n971 = local write "X=T,Y=F"(FALSE) -> ()
          }
          event "Take Single Measurement": Value Change {
            n972 = event-data() -> ()  [unwired: 1 in, 6 out]
          }
        }
      }
      frame "Stop" {
      }
      frame "Moving (old)" {
        n973 = local read "X=T,Y=F"() -> (w1481:bool)
        n974 = case shown="False" w1481 {
          tunnel: [w1512 w1514] -> w1480
          frame False {
            n975 = Absolute Value(x="Y Step Size (in)") -> (abs(x)=w1512:dbl)
          }
          frame True {
            n976 = Absolute Value(x="X Step Size (in)") -> (abs(x)=w1514:dbl)
          }
        }
        n977 = local read "Velocity"() -> (w1475:dbl)
        n978 = Multiply(x=w1475, y=1.0) -> (x*y=w1471:dbl)
        n979 = local read "Acceleration"() -> (w1470:dbl)
        n980 = Divide(x=w1475, y=w1470) -> (x/y=w1474:dbl)
        n981 = Multiply(x=w1474, y=1000.0) -> (x*y=w1472:dbl)
        n982 = disable-structure shown="Enabled" {
          disable-tunnel: w1480 -> [w1492 w1503]
          disable-tunnel: [w1487 w1495] -> w1478
          disable-tunnel: w1471 -> [w1488 w1493]
          disable-tunnel: w1472 -> [w1485 _]
          frame Enabled {
            n983 = Absolute Value(x=w1492) -> (abs(x)=w1490:dbl)
            n984 = Divide(x=w1490, y=w1488) -> (x/y=w1491:dbl)
            n985 = Multiply(x=w1491, y=1000.0) -> (x*y=w1486:dbl)
            n986 = Add(x=w1485, y=50.0) -> ()  [unwired: 1 out]
            n987 = Add(x=250.0, y=w1486) -> (x+y=w1487:dbl)
          }
          frame Disabled {
            w1499 = 10.0 ("y")
            # "Acceleration"
            n988 = Multiply(x=w1503, y=2.0) -> (x*y=w1501:dbl)
            n989 = Square(x=w1493) -> (x^2=w1504:dbl)
            n990 = Multiply(x=w1501, y=w1499) -> (x*y=w1502:dbl)
            n991 = Add(x=w1504, y=w1502) -> (x+y=w1505:dbl)
            n992 = Negate(x=w1493) -> (-x=w1508:dbl)
            n993 = Square Root(x=w1505) -> (sqrt(x)=w1507:dbl)
            n994 = Add(x=w1508, y=w1507) -> (x+y=w1506:dbl)
            n995 = Divide(x=w1506, y=w1499) -> (x/y=w1498:dbl)
            n996 = Multiply(x=w1498, y=1000.0) -> (x*y=w1496:dbl)
            n997 = Add(x=w1496, y=0.0) -> (x+y=w1495:dbl)
          }
        }
        n998 = flat-sequence {
          tunnel: w1478 -> [w1510]
          tunnel: [w1509] -> w1476
          tunnel: w1476 -> [_]
          frame #0 {
            n999 = Round Toward +Infinity(x=w1510) -> (ceil(x): smallest int >= x=w1509:dbl)
            n1000 = local write "Time to wait"(w1509) -> ()
            n1001 = property on="Moving?" class="Bool (strict)"("Val(Sgnl)"=TRUE) -> ()  [unwired: 2 in, 2 out]
          }
          frame #1 {
          }
        }
      }
      frame "Moving" {
        n1002 = flat-sequence {
          tunnel: [w1524] -> w1517
          tunnel: w1517 -> [w1532]
          frame #0 {
            n1003 = property on="Moving?" class="Bool (strict)"("Val(Sgnl)"=TRUE) -> ()  [unwired: 2 in, 2 out]
          }
          frame #1 {
            n1004 = Wait (ms)(milliseconds to wait=u32 15 ("millisecond timer value")) -> ()  [unwired: 1 out]
          }
          frame #2 {
            n1005 = property on="Read Position" class="Bool (strict)"("Val(Sgnl)"=TRUE ("Value (Signaling)")) -> ()  [unwired: 2 in, 2 out]
          }
          frame #3 {
            n1006 = while {
              stop <- w1522 stop-if-true
              n1007 = local read "Read Position"() -> (w1523:bool)
              n1008 = Not(x=w1523) -> (.not. x?=w1522:bool)
            }
          }
          frame #4 {
            n1009 = local read "X=T,Y=F"() -> (w1527:bool)
            n1010 = case shown="False" w1527 {
              tunnel: [w1528 w1530] -> w1525
              tunnel: [w1529 w1531] -> w1526
              frame False {
                n1011 = local read "Y Step Size (in)"() -> (w1528:dbl)
                n1012 = local read "Y Pos"() -> (w1529:dbl)
              }
              frame True {
                n1013 = local read "X Step Size (in)"() -> (w1530:dbl)
                n1014 = local read "X Pos"() -> (w1531:dbl)
              }
            }
            n1015 = Add(x=w1526, y=w1525) -> (x+y=w1524:dbl)
          }
          frame #5 {
            n1016 = while {
              tunnel: w1532 -> [w1538]
              stop <- w1533 stop-if-true
              n1017 = flat-sequence {
                tunnel: [w1544] -> w1535
                frame #0 {
                  n1018 = property on="Read Position" class="Bool (strict)"("Val(Sgnl)"=TRUE ("Value (Signaling)")) -> ()  [unwired: 2 in, 2 out]
                }
                frame #1 {
                  n1019 = while {
                    stop <- w1542 stop-if-true
                    n1020 = local read "Read Position"() -> (w1543:bool)
                    n1021 = Not(x=w1543) -> (.not. x?=w1542:bool)
                  }
                }
                frame #2 {
                  n1022 = local read "X=T,Y=F"() -> (w1545:bool)
                  n1023 = case shown="True" w1545 {
                    tunnel: [w1546 w1547] -> w1544
                    frame False {
                      n1024 = local read "Y Pos"() -> (w1546:dbl)
                    }
                    frame True {
                      n1025 = local read "X Pos"() -> (w1547:dbl)
                    }
                  }
                }
              }
              n1026 = Subtract(x=w1538, y=w1535) -> (x-y=w1537:dbl)
              n1027 = Absolute Value(x=w1537) -> (abs(x)=w1534:dbl)
              n1028 = Less Or Equal?(x=w1534, y=0.001) -> (x <= y?=w1533:bool)
              n1029 = flat-sequence {
                tunnel: w1533 -> [w1539]
                frame #0 {
                  n1030 = local write "Done Mov?"(w1539) -> ()
                  n1031 = Wait (ms)(milliseconds to wait=u32 5) -> ()  [unwired: 1 out]
                }
              }
            }
          }
        }
      }
    }
  }
  n1032 = while {
    shift-right: [w1553] -> _
    shift-left: "Idle" -> [w1554]
    tunnel: [w1551] -> w12
    tunnel: w18 -> [w1551]
    tunnel: [w1550] -> w11
    tunnel: w17 -> [w1550]
    tunnel: w15 -> [w1549]
    tunnel: w16 -> [w1548]
    tunnel: [w1549] -> w14
    tunnel: [w1548] -> w13
    stop <- w1552 stop-if-true
    n1033 = case shown="\"Moving\"" w1554 {
      tunnel: [w1556 "Wait" "Idle" "Idle" "Idle" "Idle" "Idle" "Idle"] -> w1553
      tunnel: [FALSE TRUE FALSE FALSE FALSE FALSE FALSE FALSE] -> w1552
      tunnel: w1551 -> [_ _ w1567 w1603 w1649 _ w1694 w1719]
      tunnel: w1550 -> [_ _ w1569 w1607 w1648 _ w1693 w1718]
      tunnel: w1549 -> [_ _ w1570 w1606 w1647 _ w1692 w1717]
      tunnel: w1548 -> [_ _ w1568 w1604 w1646 _ w1691 w1716]
      frame "Idle", Default {
        n1034 = flat-sequence {
          frame #0 {
            w1557 = FALSE
            n1035 = local write "Read Position"(w1557) -> ()
            n1036 = local write "Moving?"(w1557) -> ()
            n1037 = local write "Set Vel/Acc"(w1557) -> ()
          }
        }
        n1038 = event shown="[2] \"Read Position\": Value Change" {
          selector: _ -> [_ _ _ _ _ _ _]
          dyn-events: _ -> [_ _ _ _ _ _ _]
          timeout: _ -> [_ _ _ _ _ _ _]
          tunnel: ["Idle" "Moving" "Read Position" "Set Vel/Acc" "Stop Action" "Open Connection" "Stop"] -> w1556
          event Timeout {
            n1039 = event-data() -> ()  [unwired: 1 in, 3 out]
          }
          event "Moving?": Value Change {
            n1040 = event-data() -> ()  [unwired: 1 in, 6 out]
          }
          event "Read Position": Value Change {
            n1041 = event-data() -> ()  [unwired: 1 in, 6 out]
          }
          event "Set Vel/Acc": Value Change {
            n1042 = event-data() -> ()  [unwired: 1 in, 6 out]
          }
          event "Abort": Value Change {
            n1043 = event-data() -> ()  [unwired: 1 in, 6 out]
          }
          event "Connection": Value Change {
            n1044 = event-data() -> ()  [unwired: 1 in, 6 out]
          }
          event "Stop": Value Change {
            n1045 = event-data() -> ()  [unwired: 1 in, 6 out]
          }
        }
      }
      frame "Stop" {
      }
      frame "Moving" {
        n1046 = case shown="False" "X=T,Y=F" {
          tunnel: w1570 -> [_ w1600]
          tunnel: w1569 -> [w1574 _]
          tunnel: w1568 -> [w1586 _]
          tunnel: w1567 -> [_ w1588]
          frame False {
            n1047 = local read "Settings Y"() -> (w1581:T1)
            n1048 = Unbundle(w1581) -> ("Initial Position"=w1580:dbl, "Move Absolute/Relative Position"=w1575:dbl, "Step Delay (ms)"=w1579:u32, "Velocity (mm/s)"=w1578:dbl, "Acceleration (mm/s^2)"=w1577:dbl)  [unwired: 1 out]
            n1049 = local read "Y Step Size (in)"() -> (w1576:dbl)
            n1050 = Bundle("Y Step Size (in)"=w1576, "Initial Position"=w1580, "Move Absolute/Relative Position"=w1575, "Step Delay (ms)"=w1579, "Velocity (mm/s)"=w1578, "Acceleration (mm/s^2)"=w1577) -> (w1583:T5)  [unwired: 1 in]
            n1051 = local write "Settings Y"(w1583) -> ()
            n1052 = call "ActionEngine M2.vi"("ChannelNumber"=2, "Settings"=w1583, "SerialNumber"=w1586, "KCubeStepperControl"=w1574, "Action"=ActionEngineEnum."Step") -> ("Current Position"=w1582:dbl)  [unwired: 4 in, 1 out]
            n1053 = disable-structure shown="Disabled" {
              disable-tunnel: w1582 -> [w1587 _]
              frame Disabled {
                n1054 = local write "Y Pos"(w1587) -> ()
              }
              frame Enabled {
              }
            }
          }
          frame True {
            n1055 = local read "Settings X"() -> (w1595:T1)
            n1056 = Unbundle(w1595) -> ("Initial Position"=w1594:dbl, "Move Absolute/Relative Position"=w1589:dbl, "Step Delay (ms)"=w1593:u32, "Velocity (mm/s)"=w1592:dbl, "Acceleration (mm/s^2)"=w1591:dbl)  [unwired: 1 out]
            n1057 = local read "X Step Size (in)"() -> (w1590:dbl)
            n1058 = Bundle("X Step Size (in)"=w1590, "Initial Position"=w1594, "Move Absolute/Relative Position"=w1589, "Step Delay (ms)"=w1593, "Velocity (mm/s)"=w1592, "Acceleration (mm/s^2)"=w1591) -> (w1597:T6)  [unwired: 1 in]
            n1059 = local write "Settings X"(w1597) -> ()
            n1060 = call "ActionEngine M1.vi"("ChannelNumber"=1, "Settings"=w1597, "SerialNumber"=w1600, "KCubeStepperControl"=w1588, "Action"=ActionEngineEnum."Step") -> ("Current Position"=w1596:dbl)  [unwired: 4 in, 1 out]
            n1061 = disable-structure shown="Disabled" {
              disable-tunnel: w1596 -> [w1601 _]
              frame Disabled {
                n1062 = local write "X Pos"(w1601) -> ()
              }
              frame Enabled {
              }
            }
          }
        }
      }
      frame "Set Vel/Acc" {
        n1063 = flat-sequence {
          tunnel: [w1620] -> w1609
          tunnel: [w1612] -> w1605
          tunnel: w1609 -> [w1631]
          tunnel: [w1637] -> w1608
          tunnel: w1607 -> [w1628]
          tunnel: w1606 -> [w1636]
          tunnel: w1605 -> [w1630]
          tunnel: w1604 -> [w1633]
          tunnel: w1603 -> [w1629]
          tunnel: [w1632] -> w1602
          tunnel: w1608 -> [w1641]
          tunnel: w1602 -> [w1640]
          frame #0 {
            n1064 = local read "Settings Y"() -> (w1619:T1)
            n1065 = local read "Settings X"() -> (w1621:T1)
            n1066 = local read "Acceleration"() -> (w1613:dbl)
            n1067 = local read "Acceleration"() -> (w1627:dbl)
            n1068 = local read "Velocity"() -> (w1614:dbl)
            n1069 = local read "Velocity"() -> (w1626:dbl)
            n1070 = Unbundle(w1619) -> ("Step Size (mm)"=w1618:sgl, "Initial Position"=w1617:dbl, "Move Absolute/Relative Position"=w1616:dbl, "Step Delay (ms)"=w1615:u32)  [unwired: 2 out]
            n1071 = Unbundle(w1621) -> ("Step Size (mm)"=w1622:sgl, "Initial Position"=w1623:dbl, "Move Absolute/Relative Position"=w1624:dbl, "Step Delay (ms)"=w1625:u32)  [unwired: 2 out]
            n1072 = Bundle("Step Size (mm)"=w1618, "Initial Position"=w1617, "Move Absolute/Relative Position"=w1616, "Step Delay (ms)"=w1615, "Velocity"=w1614, "Acceleration"=w1613) -> (w1612:T7)  [unwired: 1 in]
            n1073 = Bundle("Step Size (mm)"=w1622, "Initial Position"=w1623, "Move Absolute/Relative Position"=w1624, "Step Delay (ms)"=w1625, "Velocity"=w1626, "Acceleration"=w1627) -> (w1620:T7)  [unwired: 1 in]
          }
          frame #1 {
            n1074 = local write "Settings X"(w1631) -> ()
            n1075 = local write "Settings Y"(w1630) -> ()
            n1076 = call "ActionEngine M2.vi"("ChannelNumber"=2, "Settings"=w1630, "SerialNumber"=w1633, "KCubeStepperControl"=w1628, "Action"=ActionEngineEnum."Settings") -> ("Current Position"=w1632:dbl)  [unwired: 4 in, 1 out]
            n1077 = call "ActionEngine M1.vi"("ChannelNumber"=1, "Settings"=w1631, "SerialNumber"=w1636, "KCubeStepperControl"=w1629, "Action"=ActionEngineEnum."Settings") -> ("Current Position"=w1637:dbl)  [unwired: 4 in, 1 out]
          }
          frame #2 {
            n1078 = local write "X Pos"(w1641) -> ()
            n1079 = local write "Y Pos"(w1640) -> ()
          }
        }
      }
      frame "Stop Action" {
        # "If want 2d flyover here, need to replace\nvalues after with -inf (they populate\nas 0)"
        n1080 = local read "Flyover X Linescan"() -> (w1645:bool)
        n1081 = local read "Flyover Y Linescan"() -> (w1644:bool)
        n1082 = local read "2D Flyover"() -> (w1642:bool)
        n1083 = Compound Arithmetic op=OR(w1645, w1644, w1642) -> (w1643:bool)
        n1084 = case shown="True" w1643 {
          tunnel: w1649 -> [_ w1655]
          tunnel: w1648 -> [_ w1654]
          tunnel: w1647 -> [_ w1653]
          tunnel: w1646 -> [_ w1652]
          frame False {
          }
          frame True {
            n1085 = flat-sequence {
              tunnel: w1655 -> [w1659]
              tunnel: w1654 -> [w1658]
              tunnel: w1653 -> [w1657]
              tunnel: w1652 -> [w1656]
              frame #0 {
                n1086 = local read "Settings Y"() -> (w1661:T1)
                n1087 = local read "Settings X"() -> (w1660:T1)
                n1088 = call "ActionEngine M2.vi"("ChannelNumber"=2, "Settings"=w1661, "SerialNumber"=w1656, "KCubeStepperControl"=w1658, "Action"=ActionEngineEnum."Stop Action") -> ()  [unwired: 4 in, 2 out]
                n1089 = call "ActionEngine M1.vi"("ChannelNumber"=1, "Settings"=w1660, "SerialNumber"=w1657, "KCubeStepperControl"=w1659, "Action"=ActionEngineEnum."Stop Action") -> ()  [unwired: 4 in, 2 out]
              }
              frame #1 {
                n1090 = local read "X Length"() -> (w1675:dbl)
                n1091 = local read "X Origin"() -> (w1674:dbl)
                n1092 = local read "Y Origin"() -> (w1670:dbl)
                n1093 = local read "Y Length"() -> (w1672:dbl)
                n1094 = Divide(x=w1675, y=2.0) -> (x/y=w1673:dbl)
                n1095 = Divide(x=w1672, y=2.0) -> (x/y=w1671:dbl)
                n1096 = Add(x=w1674, y=w1673) -> (x+y=w1669:dbl)
                n1097 = Add(x=w1670, y=w1671) -> (x+y=w1668:dbl)
                n1098 = local write "Y Pos"(w1668) -> ()
                n1099 = local write "X Pos"(w1669) -> ()
              }
            }
          }
        }
      }
      frame "Wait" {
        # "OLD DOES NOT DO ANYTHING"
        n1100 = while {
          tunnel: [FALSE] -> w1676
          stop <- w1681 stop-if-true
          n1101 = local read "Time"() -> (w1686:i32)
          n1102 = Tick Count (ms)() -> (millisecond timer value=w1685:u32)
          n1103 = Subtract(x=w1685, y=w1686) -> (x-y=w1683:u32)
          n1104 = Greater Or Equal?(x=w1683, y="Time to wait") -> (x >= y?=w1681:bool)
          "Done Mov?" <- w1681
        }
        n1105 = flat-sequence {
          tunnel: w1676 -> [w1680]
          frame #0 {
            n1106 = local write "Move Y (in)"(w1680) -> ()
            n1107 = local write "Move X (in)"(w1680) -> ()
          }
        }
        n1108 = flat-sequence {
          frame #0 {
            n1109 = Tick Count (ms)() -> (millisecond timer value=→"Time":u32)
          }
        }
      }
      frame "Read Position" {
        n1110 = flat-sequence {
          tunnel: w1691 -> [w1697]
          tunnel: w1692 -> [w1698]
          tunnel: w1693 -> [w1699]
          tunnel: w1694 -> [w1700]
          tunnel: [w1700] -> w1690
          tunnel: [w1699] -> w1689
          tunnel: [w1698] -> w1688
          tunnel: [w1697] -> w1687
          tunnel: w1690 -> [w1706]
          tunnel: w1689 -> [w1705]
          tunnel: w1688 -> [w1704]
          tunnel: w1687 -> [w1703]
          frame #0 {
          }
          frame #1 {
            n1111 = local read "Settings X"() -> (w1710:T1)
            n1112 = local read "Settings Y"() -> (w1709:T1)
            n1113 = call "ActionEngine M2.vi"("ChannelNumber"=2, "Settings"=w1709, "SerialNumber"=w1703, "KCubeStepperControl"=w1705, "Action"=ActionEngineEnum."Get Position") -> ("Current Position"=w1702:dbl)  [unwired: 4 in, 1 out]
            n1114 = call "ActionEngine M1.vi"("ChannelNumber"=1, "Settings"=w1710, "SerialNumber"=w1704, "KCubeStepperControl"=w1706, "Action"=ActionEngineEnum."Get Position") -> ("Current Position"=w1701:dbl)  [unwired: 4 in, 1 out]
            n1115 = local write "Y Pos"(w1702) -> ()
            n1116 = local write "X Pos"(w1701) -> ()
          }
          frame #2 {
            n1117 = local write "Read Position"(FALSE ("Read Position")) -> ()
          }
        }
      }
      frame "Open Connection" {
        n1118 = local read "Settings X"() -> (w1715:T1)
        n1119 = local read "Settings Y"() -> (w1714:T1)
        n1120 = call "ActionEngine M2.vi"("ChannelNumber"=2, "Settings"=w1714, "SerialNumber"=w1716, "KCubeStepperControl"=w1718, "Action"=ActionEngineEnum."Open Connection") -> ()  [unwired: 4 in, 2 out]
        n1121 = call "ActionEngine M1.vi"("ChannelNumber"=1, "Settings"=w1715, "SerialNumber"=w1717, "KCubeStepperControl"=w1719, "Action"=ActionEngineEnum."Open Connection") -> ()  [unwired: 4 in, 2 out]
      }
    }
  }
  n1122 = Close Python Session(session in=w19) -> ()  [unwired: 1 in, 1 out]
  n1123 = flat-sequence {
    tunnel: w14 -> [w1729]
    tunnel: w13 -> [w1726]
    tunnel: w12 -> [w1728]
    tunnel: w11 -> [w1727]
    tunnel: [w1727] -> w2
    tunnel: [w1726] -> w1
    tunnel: w2 -> [w1734]
    tunnel: w1 -> [w1733]
    frame #0 {
      n1124 = local read "Settings X"() -> (w1732:T1)
      n1125 = call "ActionEngine M1.vi"("ChannelNumber"=1, "Settings"=w1732, "SerialNumber"=w1729, "KCubeStepperControl"=w1728, "Action"=ActionEngineEnum."Close Connection") -> ()  [unwired: 4 in, 2 out]
    }
    frame #1 {
      n1126 = local read "Settings Y"() -> (w1737:T1)
      n1127 = call "ActionEngine M2.vi"("ChannelNumber"=2, "Settings"=w1737, "SerialNumber"=w1733, "KCubeStepperControl"=w1734, "Action"=ActionEngineEnum."Close Connection") -> ()  [unwired: 4 in, 2 out]
    }
    frame #2 {
      n1128 = local write "Stop"(FALSE ("Stop")) -> ()
    }
  }
